vi "Text control 2 v2.3.vi"() -> ()   [LabVIEW 2016]
panel:
  out "Total lines":i32
  out "Line running":i32
  in  "byte count":u32=64
  in  "Serial Settings:Serial End Mode for Reads":u16(ring)=2 items=["None", "LastBit", "TermChar"]
  in  "Timeout (ms)":u32=10000
  in  "Enable Termination\nChar (T)":bool=TRUE
  in  "Termination char\n(0xA = '\\n' = LF)\n(0xD = '\\r' = CR)":u8=13 format="%.0x"
  in  "flow control":u16(ring) items=["None"=0, "XON/XOFF"=1, "RTS/CTS"=2, "DTR/DSR"=4]
  in  "stop bits":u16(ring)=10 items=["1.0"=10, "1.5"=15, "2.0"=20]
  in  "parity":u16(ring) items=["None", "Odd", "Even", "Mark", "Space"]
  in  "data bits":u16=8 min=5 max=8 step=1
  in  "VISA resource name":refnum<visa-resource-name>="COM6"
  in  "baud rate":u32=9600
  out "Serial output":string
  out "error out":errorcluster
  in  "Units":bool
  out "Elapsed Time":dbl caption="Elapsed Time (s)"
  out "Ion vs time":cluster{"Y data in":dbl[], "X data in":dbl[]}[](graph)
  out "Ig":dbl format="%.2e"
  out "Id":dbl format="%.2e"
  out "Is":dbl format="%.2e"
  out "I vs Vg":cluster{"Y data in":dbl[], "X data in":dbl[]}[](graph)
  in  "Panel Controls 2":T1={"Emergency Stop"=refnum, "TransGraph Max"=1e-05, "Text/Graph (text=false)"=TRUE, "TransGraph Min"=1e-11} {"TransGraph Min" format="%.2e"; "TransGraph Max" format="%.2e"}
  out "Command running:":string="#output s 0 0 0 -0.008 0.008 0.002"
  in  "Standby":T2
  in  "Full Reset":bool
  in  "SMU4":cluster{"on/off":bool, "Voltage":dbl} {"Voltage" min=-100.0 max=100.0 format="%.2f"}
  in  "Source/Drain Range":u8(slide)=6 max=11 scale=0.0..11.0
  in  "Source/Drain\nRange mode":u16(ring) items=["Auto", "Limited", "Fixed"]
  in  "Gate Range":u8(slide)=6 max=11 scale=0.0..11.0
  in  "Gate Range\nmode":u16(ring) items=["Auto", "Limited", "Fixed"]
  in  "Gate":T3={"Gate Start"=0.0, "Gate Stop"=2.0, "Gate Step (linear only)"=1.0, "Gate Compliance"=0.0001, "Gate PComp"=0.0, "Range mode"=0, "Range"=6} {"Range" max=11 scale=0.0..11.0; "Range mode" items=["Auto", "Limited", "Fixed"]; "Gate PComp" format="%^.2e"; "Gate Compliance" format="%^.2e"; "Gate Step (linear only)" format="%^.4e"; "Gate Stop" format="%^.4e"; "Gate Start" format="%^.4e"}
  in  "Drain 2":T4={"Drain Start"=0.0, "Drain Stop"=2.0, "Drain Compliance"=0.0001, "Drain Step"=1.0, "Drain PComp"=0.0, "Range mode"=0, "Range"=6} {"Range" max=11 scale=0.0..11.0; "Range mode" items=["Auto", "Limited", "Fixed"]; "Drain PComp" format="%^.2e"; "Drain Step" format="%^.4e"; "Drain Compliance" format="%^.2e"; "Drain Stop" format="%^.4e"; "Drain Start" format="%^.4e"}
  in  "Timings 2":T5={"integration time"=0, "Short/Long integration time"=0.00064, "hold time (sec)"=0.0, "delay time (sec)"=0.0, "Step Time (0 disables)"=0.0, "sweep method"=0, "Pulse period"=0.005, "Base voltage"=0.0, "Pulse width"=0.0005} {"Pulse width" min=0.0005 max=0.1 step=0.0001 format="%.4f"; "Base voltage" format="%^.4e"; "Pulse period" min=0.005 max=1.0 step=0.0001 format="%.4f"; "sweep method" items=["Continuous", "Pulsed"]; "Step Time (0 disables)" format="%.2f"; "delay time (sec)" format="%.4f"; "hold time (sec)" format="%.4f"; "Short/Long integration time" format="%^.0e"; "integration time" scale=0.0..2.0}
  in  "Panel Controls":T6={"Emergency Stop"=refnum, "TransGraph Max"=1e-05, "Text/Graph (text=false)"=TRUE} {"TransGraph Max" format="%.2e"}
  in  "Interrupt run":bool
  in  "Drain: Compliance":dbl=0.001 format="%.8f"
  in  "Gate: Compliance":dbl=0.001 format="%.8f"
  out "Path":path=path "C:/users/rlp38/09Apr2009LTtesting/test2.txt"
  in  "hold time /s":dbl format="%.2f"
  in  "delay time /s":dbl format="%.2f"
  in  "integration time":u32(slide) max=2 step=1 scale=0.0..2.0
  in  "Integration time (short)":dbl=0.0019 min=8e-05 max=0.0019 step=8e-05 format="%^.0e"
  in  "Integration time (long)":dbl=0.32 min=0.04 max=2.0 step=0.02 format="%.2f"
  in  "Step delay /s":dbl format="%.2f"
  in  "Program":string="#pulsedstressV d 0.03 20 0 0.5 0.0827 5\n#\n#itime s\n#gaterangemode l\n#drainrangemode l\n#pulsed on 0.05 0 0.02\n#transfer d 1 -1 -0.1 -1 -1 0\n#wait-min 1\n#transfer d 1 -1 -0.1 -1 -1 0\n#output d 0 -1 -0.5 0 -1 -0.1\n#transfer d -10 40 1 5 40 35\n#transfer d -10 40 1 5 40 35\n#output d 0 40 20 0 40 1\n#\n#\n#sample 1 0.008 221 6 0.003\n#samplei 400e-6 200 6 0.002 0.1\n#vsu2pulse -10 4\n#\n#stressV 0.016 0.03 2e-4 0.1e-3 11\n#stressI 220e-7 0.08 15\n#transfer s -1 1 0.5 -0.005 0.005 0.005\n#output s 0 0 0 -0.008 0.008 0.002\n"
  # "Syntax:\nitime [s|m|l]\ngaterangemode [a|l|f]\ndrainrangemode [a|l|f]\npulsed [on|off] PulsePeriod(sec) PulseBaseVoltage PulseONWidth(sec)\nstandby [on l off]\nwait NumMilliseconds\nwait-min NumMinutes\n# texthere = comment\ntransfer [s|d] VgStart VgStop VgStep VdStart VdStop VdStep\noutput [s|d] VgStart VgStop VgStep VdStart VdStop VdStep\nsample Vg Vd NumSamples Time(s) SampleInterval(s)\nsamplei Idg NumSamples Time(s) SampleInterval(s) VDGcompliance\n# if in doubt use SampleInterval(s) = 0.004\nstressV VG VD IGcompliance IDcompliance Duration(sec)\nstressI IDG VDGcompliance Duration(sec)\nvsu2pulse Bias Duration(s)\npulsedstressV [s|d] VEstop VgON VgOFF Period(s) PulseONwidth(s) Vd\nsample-fpp Vg Vd NumSamples Time\nresample-fpp Vg Vd\ntransfer-fpp [s|d] VgStart VgStop VgStep VdStart VdStop VdStep\noutput-fpp [s|d] VgStart VgStop VgStep VdStart VdStop VdStep\nserial SerialPortCommand"
  # "Time"
  # "Sec"
  # "Min"
  # "100 samples is approx 13s with medium integration"
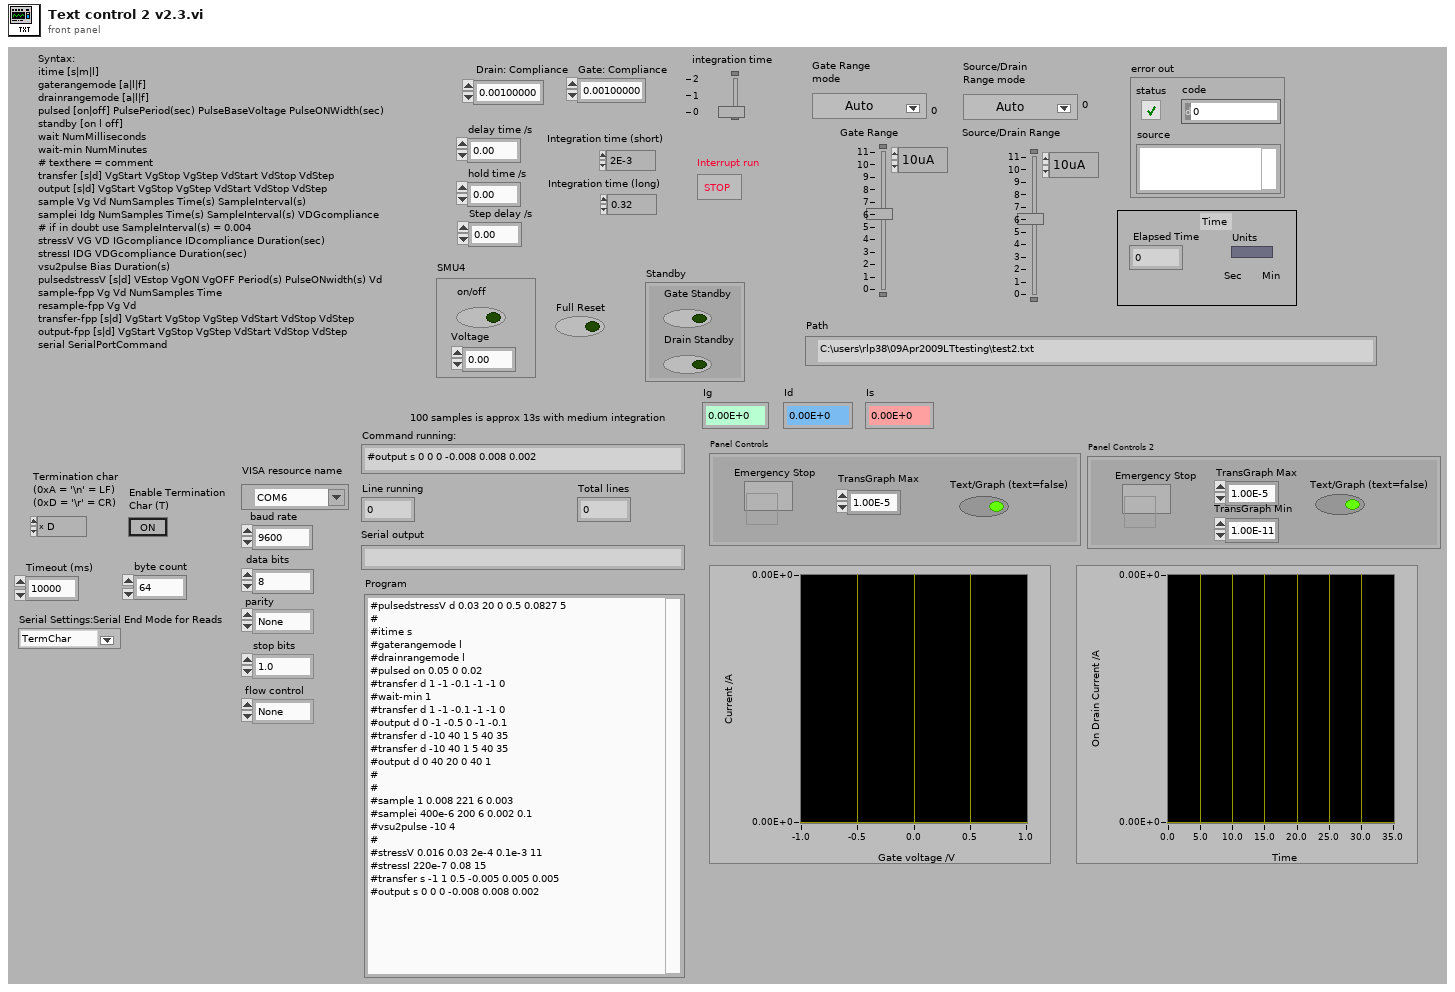
[diagram p1: front panel]
types:
  T1 = cluster{"Emergency Stop":refnum<vi>, "TransGraph Max":dbl, "Text/Graph (text=false)":bool, "TransGraph Min":dbl}
  T2 = cluster{"Gate Standby":bool, "Drain Standby":bool}
  T3 = cluster{"Gate Start":dbl, "Gate Stop":dbl, "Gate Step (linear only)":dbl, "Gate Compliance":dbl, "Gate PComp":dbl, "Range mode":u16, "Range":u8}
  T4 = cluster{"Drain Start":dbl, "Drain Stop":dbl, "Drain Compliance":dbl, "Drain Step":dbl, "Drain PComp":dbl, "Range mode":u16, "Range":u8}
  T5 = cluster{"integration time":u32, "Short/Long integration time":dbl, "hold time (sec)":dbl, "delay time (sec)":dbl, "Step Time (0 disables)":dbl, "sweep method":u16, "Pulse period":dbl, "Base voltage":dbl, "Pulse width":dbl}
  T6 = cluster{"Emergency Stop":refnum<vi>, "TransGraph Max":dbl, "Text/Graph (text=false)":bool}
  T7 = enum16{"open", "replace", "create", "open or create", "replace or create", "replace or create with confirmation"}
  T8 = cluster{"V2 Start":dbl, "V2 Step":dbl, "Number of points":i32}
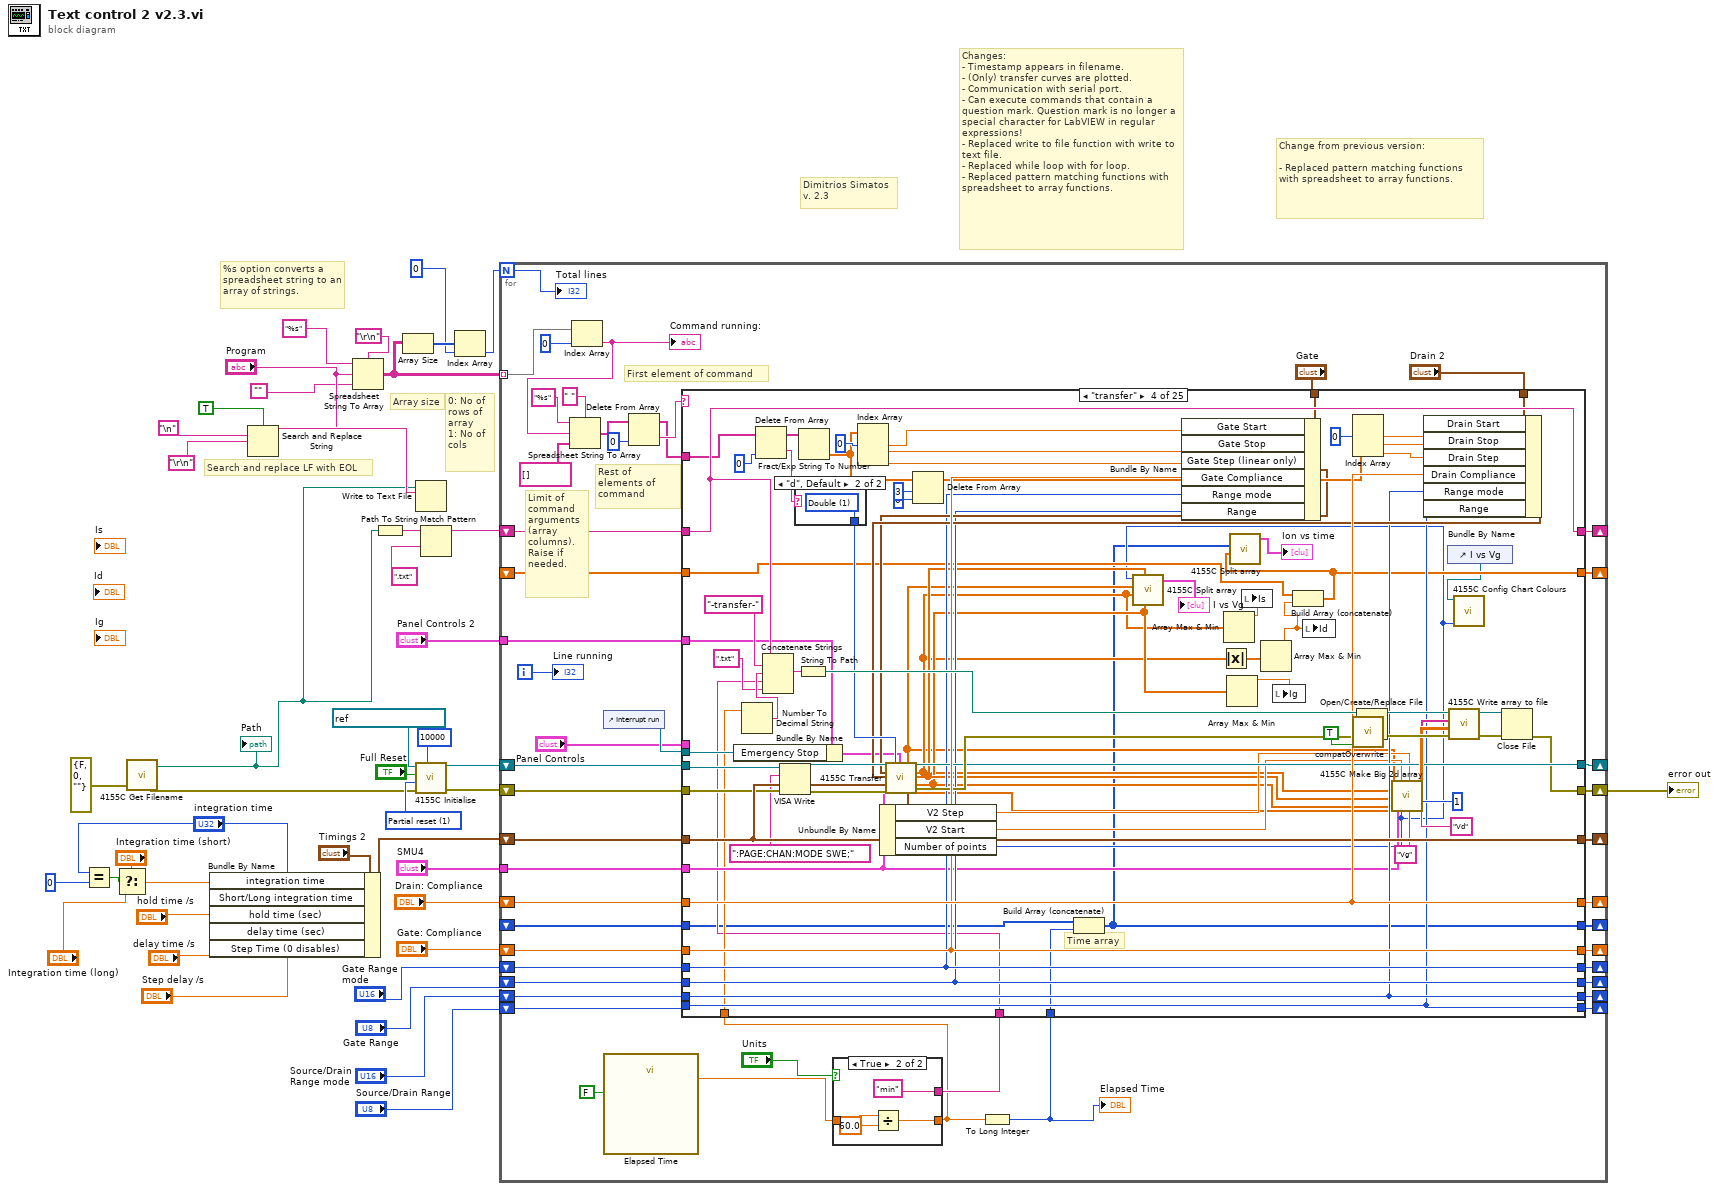
[diagram p0: block diagram]
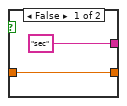
[diagram p2: hidden frame]
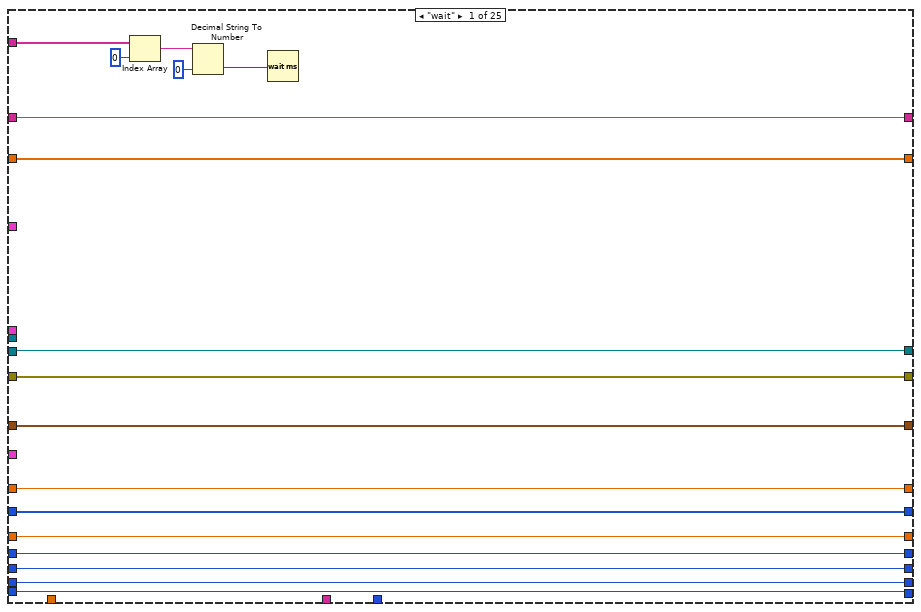
[diagram p3: hidden frame]
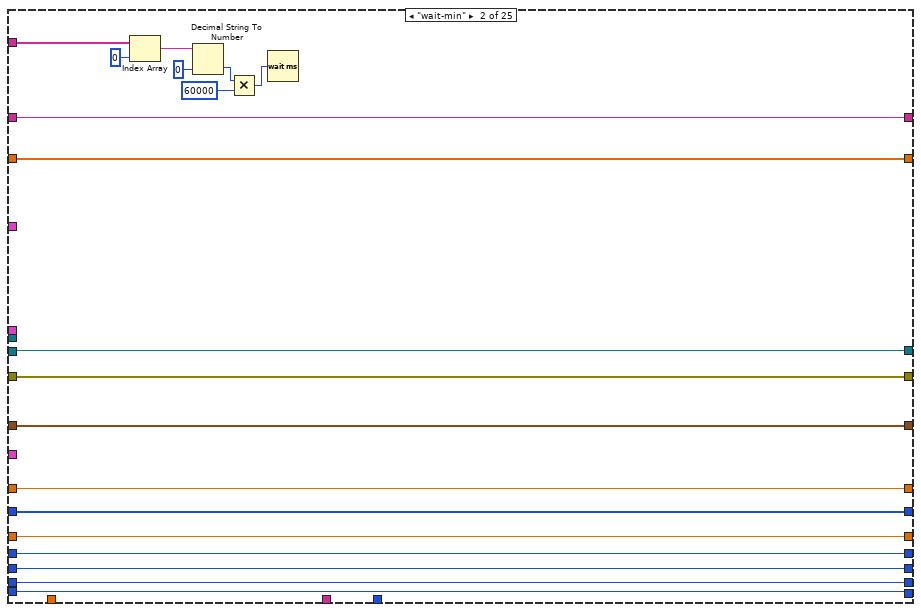
[diagram p4: hidden frame]
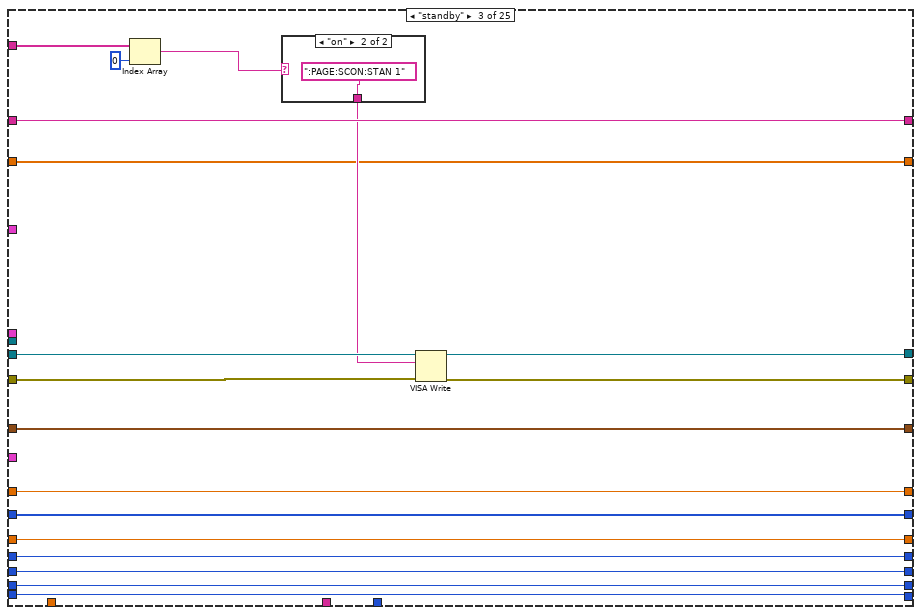
[diagram p5: hidden frame]
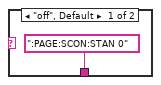
[diagram p6: hidden frame]
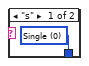
[diagram p7: hidden frame]
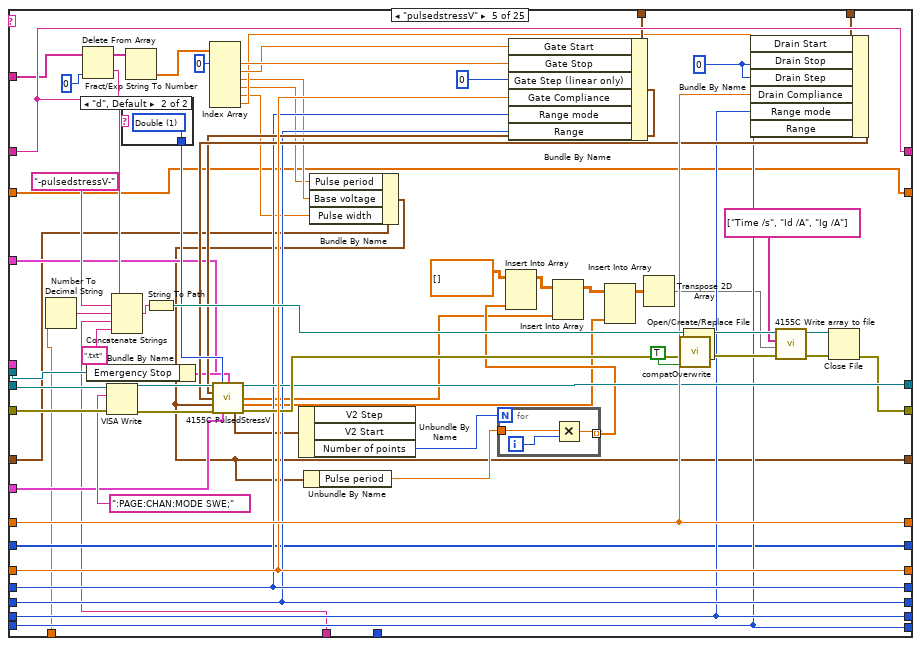
[diagram p8: hidden frame]
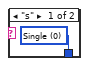
[diagram p9: hidden frame]
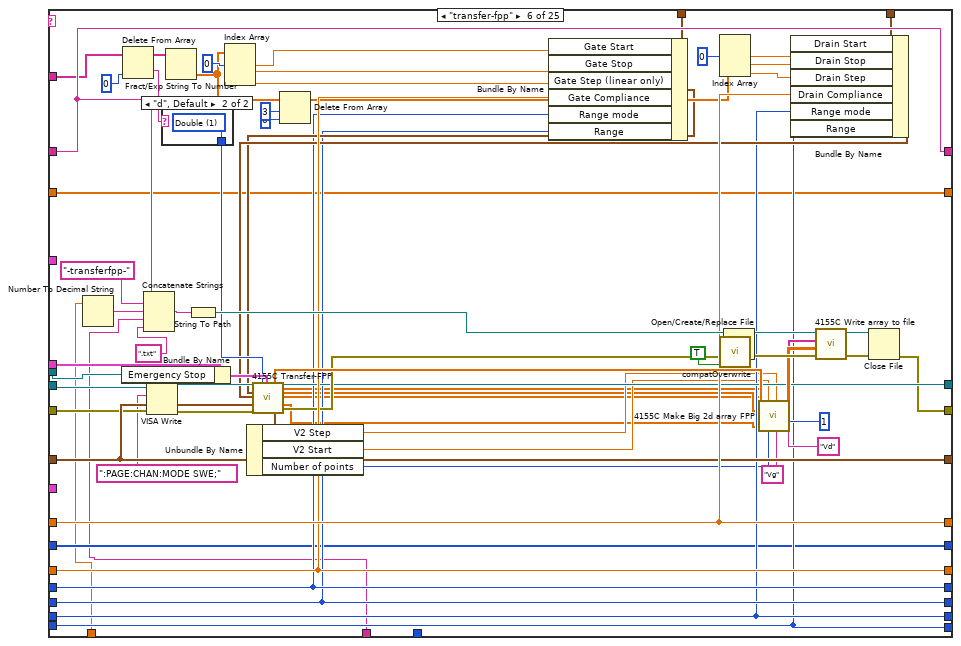
[diagram p10: hidden frame]
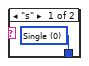
[diagram p11: hidden frame]
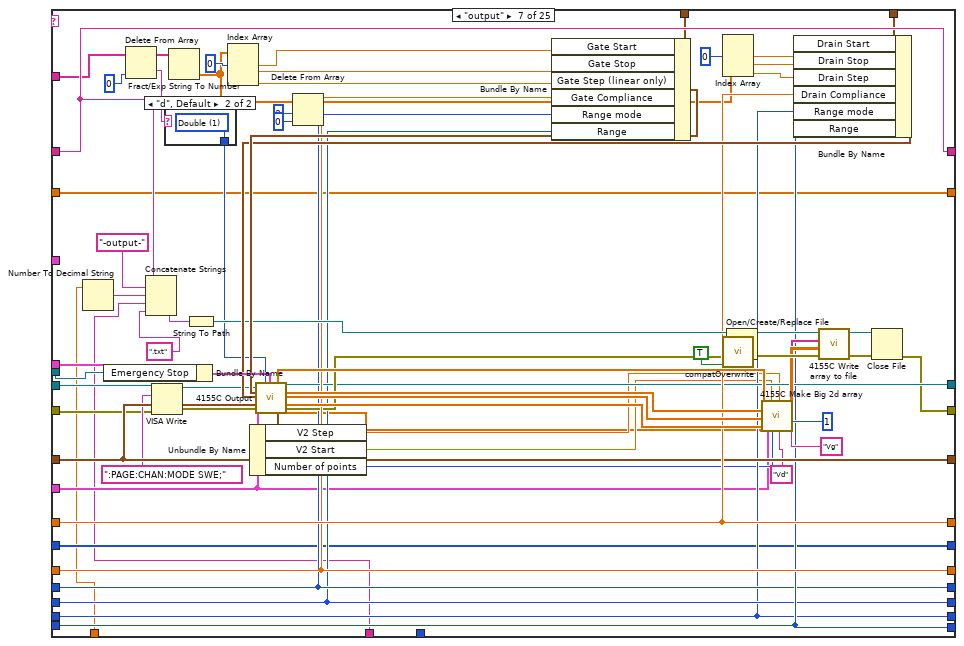
[diagram p12: hidden frame]
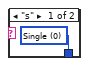
[diagram p13: hidden frame]
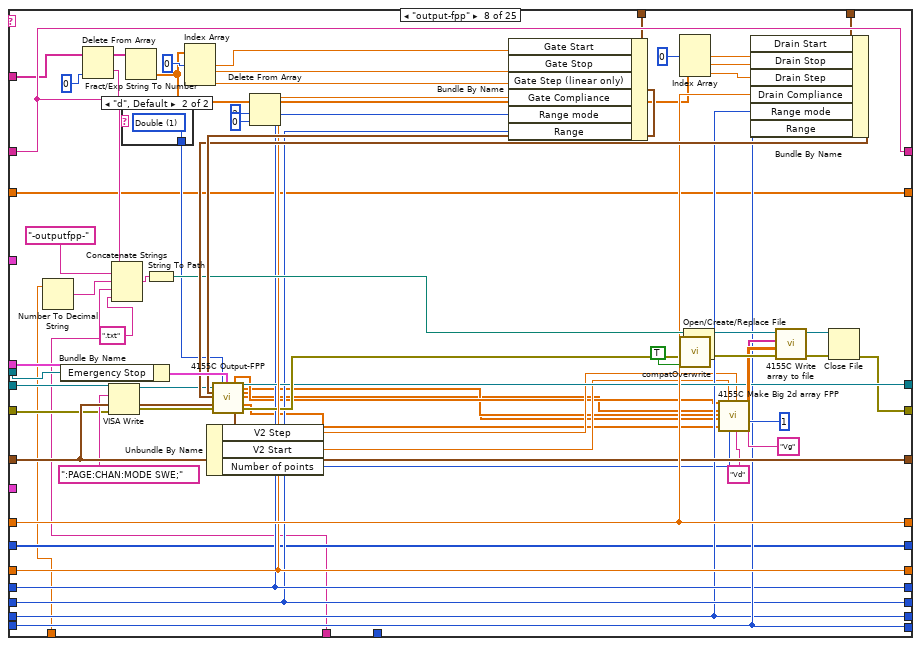
[diagram p14: hidden frame]
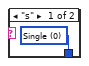
[diagram p15: hidden frame]
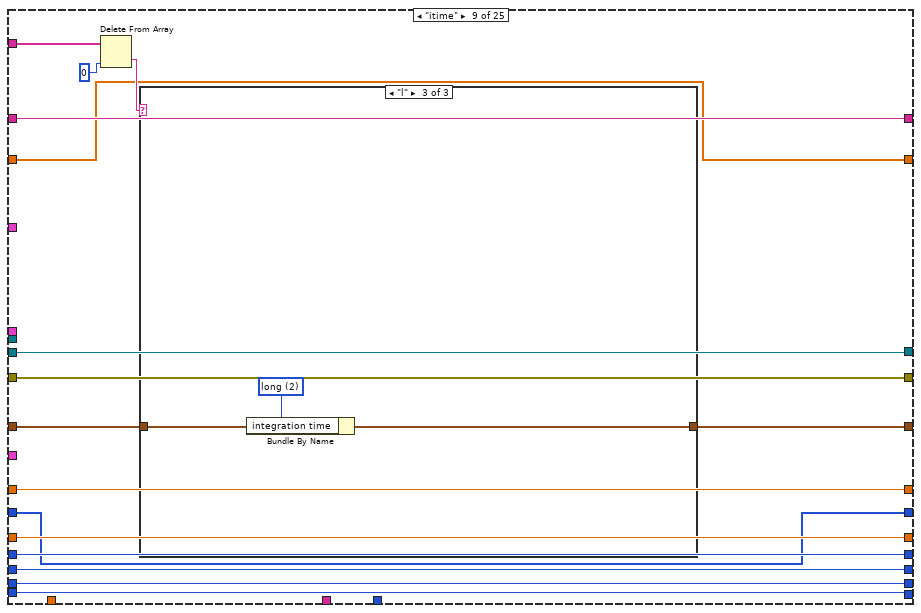
[diagram p16: hidden frame]
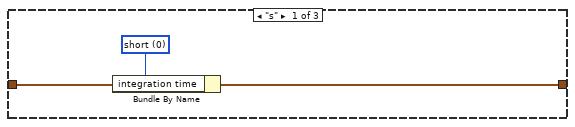
[diagram p17: hidden frame]
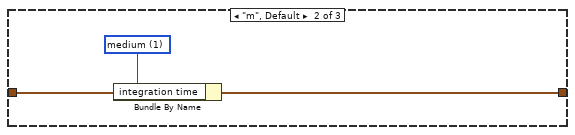
[diagram p18: hidden frame]
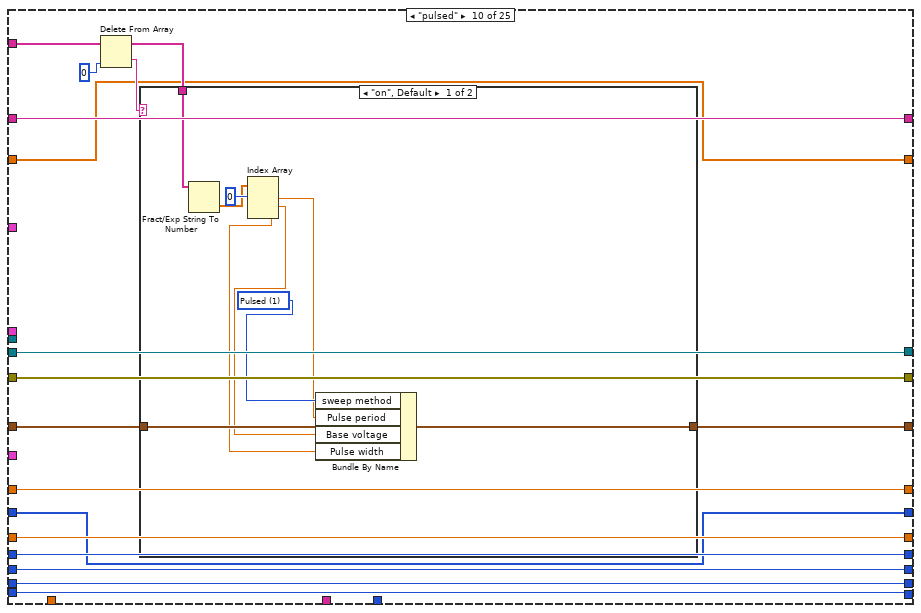
[diagram p19: hidden frame]
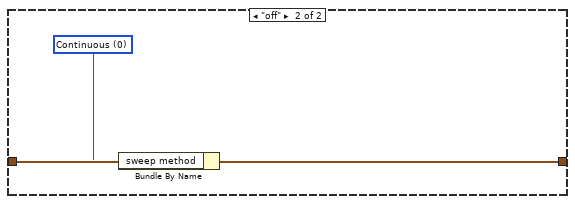
[diagram p20: hidden frame]
diagram:
  w35 = u16 1 items=["Reset All", "Partial reset"] ("Type of reset")
  # "Array size"
  # "%s option converts a spreadsheet string to an array of strings."
  # "0: No of rows of array\n1: No of cols"
  # "Change from previous version:\n\n- Replaced pattern matching functions with spreadsheet to array functions."
  # "Dimitrios Simatos\nv. 2.3"
  # "Changes:\n- Timestamp appears in filename.\n- (Only) transfer curves are plotted.\n- Communication with serial port.\n- Can execute commands that contain a question mark. Question mark is no longer a special character for LabVIEW in regular expressions!\n- Replaced write to file function with write to text file.\n- Replaced while loop with for loop.\n- Replaced pattern matching functions with spreadsheet to array functions."
  # "Search and replace LF with EOL"
  n1 = Equal?(x="integration time", y=u32 0) -> (x = y?=w39:bool)
  n2 = Select(t="Integration time (short)", s=w39, f="Integration time (long)") -> (s? t:f=w43:dbl)
  n3 = call "4155C Get Filename.vi"("error in (no error)"=errorcluster {"status"=FALSE, "code"=0, "source"=""}) -> ("error out"=w30:errorcluster, "path"=w1:path)  [unwired: 2 in, 1 out]
  "Path" <- w1
  n4 = Bundle By Name(cluster="Timings 2", "integration time"="integration time", "Short/Long integration time"=w43, "hold time (sec)"="hold time /s", "delay time (sec)"="delay time /s", "Step Time (0 disables)"="Step delay /s") -> (w27:T5)
  n5 = Search and Replace String(replace all?=TRUE ("replace all? (F)"), input string="Program", search string="\n", replace string="\r\n") -> (result string=w17:string)  [unwired: 4 in, 3 out]
  n6 = Spreadsheet String To Array(delimiter (Tab)="\r\n", format string="%s", spreadsheet string="Program", array type (2D Dbl)="") -> (array=w7:string[][])
  n7 = Path To String(path=w1) -> (string=w4:string)
  n8 = Array Size(array=w7) -> (size(s)=w11:i32[])
  n9 = Write to Text File(file (use dialog)=w1, text=w17) -> ()  [unwired: 2 in, 3 out]
  n10 = call "4155C Initialise.vi"("VISA resource name in"=refnum<visa-resource-name> "GPIB0::14::INSTR", "Reset"="Full Reset", "Type of reset"=w35, "error in (no error)"=w30, "VISA Timeout Value"=u32 10000) -> ("VISA Resource Name out"=w29:refnum<visa-resource-name>, "error out"=w28:errorcluster)
  n11 = Match Pattern(string=w4, regular expression=".txt") -> (before substring=w2:string)  [unwired: 1 in, 3 out]
  n12 = Index Array(array=w11, index=0) -> (element=w9:i32)
  n13 = for {
    N: w9 -> [w53]
    tunnel: "SMU4" -> [w68]
    shift-left: "Source/Drain Range" -> [w73]
    shift-right: [w69] -> _
    shift-left: "Source/Drain\nRange mode" -> [w74]
    shift-right: [w70] -> _
    shift-left: "Gate Range" -> [w75]
    shift-right: [w71] -> _
    shift-left: "Gate Range\nmode" -> [w76]
    shift-right: [w72] -> _
    shift-left: "Gate: Compliance" -> [w87]
    shift-right: [w82] -> _
    shift-left: "Drain: Compliance" -> [w88]
    shift-right: [w83] -> _
    shift-left: w27 -> [w89]
    shift-right: [w84] -> _
    shift-left: w28 -> [w90]
    shift-right: [w85] -> w13
    shift-left: w29 -> [w91]
    shift-right: [w86] -> _
    shift-left: w2 -> [w92]
    shift-right: [w81] -> _
    tunnel: "Panel Controls 2" -> [w67]
    shift-right: [w66] -> _
    shift-left: _ -> [w65]
    shift-right: [w60] -> _
    shift-left: _ -> [w59]
    tunnel: w7 -> [w56] mode=indexing
    i -> [w54]
    # "Limit of command arguments (array columns). Raise if needed."
    # "Rest of elements of command"
    # "First element of command"
    n14 = Index Array(array=w56, index=0 ("line index")) -> (element=w49:string)
    "Command running:" <- w49
    n15 = Spreadsheet String To Array(delimiter (Tab)=" ", format string="%s", spreadsheet string=w49, array type (2D Dbl)=string[] []) -> (array=w46:string[])
    n16 = control-ref of="Interrupt run"() -> (w80:refnum<vi>)
    n17 = call "Elapsed Time"("Auto Reset"=FALSE) -> ("Elapsed Time (s)"=w61:dbl)  [unwired: 11 in, 7 out]
    n18 = Delete From Array(array=w46, index=0) -> (deleted portion=w47:string, array with subset deleted=w45:string[])  [unwired: 1 in]
    n19 = case shown="True" "Units" {
      tunnel: ["sec" "min"] -> w62
      tunnel: [w93 w97] -> w58
      tunnel: w61 -> [w93 w96]
      frame False {
      }
      frame True {
        n20 = Divide(x=w96, y=60.0) -> (x/y=w97:dbl)
      }
    }
    n21 = To Long Integer(number=w58) -> (32bit integer=w57:i32)
    "Elapsed Time" <- w57
    n22 = case shown="\"transfer\"" w47 {
      tunnel: w45 -> [w115 w134 w152 w216 w287 w356 w423 w498 w536 w562 w589 w614 w635 w649 _ _ w753 w814 _ w879 w923 w965 w1035 w1097 w1104]
      tunnel: w92 -> [w110 w130 w150 w224 w294 w364 w431 w506 w525 w551 w581 w607 w629 w642 w661 w703 w731 w796 w827 w866 w910 w953 w1029 w1093 w1106]
      tunnel: w91 -> [w109 w129 w141 w194 w278 w333 w399 w474 w526 w552 w582 w608 w630 w643 w666 w705 w759 w820 w831 w885 w929 w971 w1041 w1051 w1110]
      tunnel: w90 -> [w108 w128 w140 w193 w277 w332 w396 w471 w527 w553 w583 w609 w631 w644 w665 w676 w758 w819 w830 w884 w928 w970 w1040 w1050 w1109]
      tunnel: w89 -> [w107 w127 w149 w220 w253 w360 w427 w502 w535 w561 w580 w606 w628 w641 w664 w700 w722 w788 w836 w859 w903 w946 w1028 w1092 w1111]
      tunnel: w88 -> [w106 w126 w148 w222 w292 w362 w429 w504 w534 w560 w588 w613 w634 w648 w663 w685 w757 w818 w839 w883 w927 w969 w1039 w1101 w1112]
      tunnel: w87 -> [w105 w125 w147 w221 w291 w361 w428 w503 w533 w559 w587 w612 w633 w647 w662 w686 w732 w797 w838 w867 w911 w954 w1030 w1094 w1114]
      tunnel: [w109 w129 w139 w218 w289 w358 w425 w500 w526 w552 w582 w608 w630 w643 w666 w705 w723 w770 w829 w860 w904 w947 w981 w1053 w1110] -> w86
      tunnel: [w108 w128 w138 w217 w288 w357 w424 w499 w527 w553 w583 w609 w631 w644 w665 w675 w733 w771 w828 w868 w912 w955 w980 w1052 w1108] -> w85
      tunnel: [w107 w127 w149 w220 w249 w360 w427 w502 w528 w554 w580 w606 w628 w641 w664 w700 w722 w788 w836 w859 w903 w946 w1028 w1092 w1111] -> w84
      tunnel: [w106 w126 w148 w222 w292 w362 w429 w504 w534 w560 w588 w613 w634 w648 w663 w685 w757 w818 w839 w883 w927 w969 w1039 w1101 w1112] -> w83
      tunnel: [w105 w125 w147 w221 w291 w361 w428 w503 w533 w559 w587 w612 w633 w647 w662 w686 w732 w797 w838 w867 w911 w954 w1030 w1094 w1114] -> w82
      tunnel: [w110 w130 w150 w224 w294 w364 w431 w506 w525 w551 w581 w607 w629 w642 w661 w703 w731 w796 w827 w866 w910 w953 w1029 w1093 w1106] -> w81
      tunnel: w80 -> [_ _ _ w227 w298 w369 w439 w510 _ _ _ _ _ _ _ _ w728 w793 _ w865 w909 w952 w1001 w1069 _]
      tunnel: "Gate" -> [_ _ _ w203 w281 w343 w410 w485 _ _ _ _ _ _ _ _ _ _ _ _ _ _ _ _ _]
      tunnel: "Drain 2" -> [_ _ _ w202 w280 w342 w409 w484 _ _ _ _ _ _ _ _ _ _ _ _ _ _ _ _ _]
      tunnel: "Panel Controls" -> [_ _ _ _ _ w341 w408 w483 _ _ _ _ _ _ _ _ _ _ _ _ _ _ _ _ _]
      tunnel: w76 -> [w104 w124 w146 w187 w271 w326 w394 w469 w532 w558 _ w605 w627 w640 w660 w687 w718 w784 w832 w855 w899 w942 w1024 w1088 w1115]
      tunnel: w75 -> [w103 w123 w145 w186 w270 w325 w393 w468 w531 w557 w586 _ w618 w646 w659 w688 w719 w785 w833 w856 w900 w943 w1025 w1089 w1116]
      tunnel: w74 -> [w102 w122 w144 w185 w269 w324 w392 w467 w530 w556 w585 w611 w632 _ w658 w689 w720 w786 w834 w857 w901 w944 w1026 w1090 w1117]
      tunnel: w73 -> [w101 w121 w143 w184 w268 w323 w395 w470 w529 w555 w584 w610 _ w645 w657 w690 w721 w787 w835 w858 w902 w945 w1027 w1091 w1118]
      tunnel: [w104 w124 w146 w187 w271 w326 w394 w469 w532 w558 w579 w605 w627 w640 w660 w687 w718 w784 w832 w855 w899 w942 w1024 w1088 w1115] -> w72
      tunnel: [w103 w123 w145 w186 w270 w325 w393 w468 w531 w557 w586 w597 w618 w646 w659 w688 w719 w785 w833 w856 w900 w943 w1025 w1089 w1116] -> w71
      tunnel: [w102 w122 w144 w185 w269 w324 w392 w467 w530 w556 w585 w611 w632 w639 w658 w689 w720 w786 w834 w857 w901 w944 w1026 w1090 w1117] -> w70
      tunnel: [w101 w121 w143 w184 w268 w323 w395 w470 w529 w555 w584 w610 w619 w645 w657 w690 w721 w787 w835 w858 w902 w945 w1027 w1091 w1118] -> w69
      tunnel: w68 -> [_ _ _ w179 w265 _ w387 _ _ _ _ _ _ _ _ _ _ _ _ _ _ _ _ _ _]
      tunnel: w67 -> [_ _ _ w177 w264 _ _ _ _ _ _ _ _ _ _ _ _ _ _ _ _ _ _ _ _]
      tunnel: [w100 w117 w136 w166 w241 w313 w384 w456 w524 w549 w578 w596 w617 w638 w656 w671 w710 w768 w826 w844 w892 w936 w978 w1046 w1107] -> w66
      tunnel: w65 -> [w100 w117 w136 w165 w241 w313 w384 w456 w524 w549 w578 w596 w617 w638 w656 w671 w710 w768 w826 w844 w892 w936 w978 w1046 w1107]
      tunnel: w58 -> [_ _ _ w161 w238 w311 w381 w453 _ _ _ _ _ _ _ w669 w708 w765 _ w841 w889 w933 w975 w1042 _]
      tunnel: w62 -> [_ _ _ w158 w237 w309 w380 w452 _ _ _ _ _ _ _ w667 w706 w764 _ w840 w888 w932 w974 w1043 _]
      tunnel: w57 -> [_ _ _ w155 _ _ _ _ _ _ _ _ _ _ _ _ _ _ _ _ _ _ _ _ _]
      tunnel: [w99 w116 w135 w157 w240 w312 w383 w455 w523 w548 w577 w595 w616 w637 w655 w670 w709 w767 w825 w843 w891 w935 w977 w1045 w1113] -> w60
      tunnel: w59 -> [w99 w116 w135 w156 w240 w312 w383 w455 w523 w548 w577 w595 w616 w637 w655 w670 w709 w767 w825 w843 w891 w935 w977 w1045 w1113]
      frame "wait" {
        n23 = Index Array(array=w115, index=0 ("Index")) -> (element=w113:string)
        n24 = Decimal String To Number(string=w113, default (0L)=u32 0) -> (number=w112:u32)  [unwired: 1 in, 1 out]
        n25 = Wait (ms)(milliseconds to wait=w112) -> ()  [unwired: 1 out]
      }
      frame "wait-min" {
        n26 = Index Array(array=w134, index=0 ("Index")) -> (element=w132:string)
        n27 = Decimal String To Number(string=w132, default (0L)=u32 0) -> (number=w120:u32)  [unwired: 1 in, 1 out]
        n28 = Multiply(x=w120, y=u32 60000) -> (x*y=w119:u32)
        n29 = Wait (ms)(milliseconds to wait=w119) -> ()  [unwired: 1 out]
      }
      frame "standby" {
        n30 = Index Array(array=w152, index=0 ("Index")) -> (element=w142:string)
        n31 = case shown="\"on\"" w142 {
          tunnel: [":PAGE:SCON:STAN 0" ":PAGE:SCON:STAN 1"] -> w137
          frame "off", Default {
          }
          frame "on" {
          }
        }
        n32 = VISA Write(VISA resource name=w141, write buffer=w137, error in (no error)=w140) -> (VISA resource name out=w139:refnum<visa-resource-name>, error out=w138:errorcluster)  [unwired: 1 out]
      }
      frame "transfer" {
        # "Time array"
        n33 = Bundle By Name(cluster=w177, "Emergency Stop"=w227) -> (w178:T1)
        n34 = Number To Decimal String(number=w161) -> (decimal integer string=w160:string)  [unwired: 1 in]
        n35 = Delete From Array(array=w216, index=0 ("Index")) -> (deleted portion=w214:string, array with subset deleted=w213:string[])  [unwired: 1 in]
        n36 = Concatenate Strings(w224, "-transfer-" ("Prefix"), w160, w158, ".txt" ("Suffix")) -> (w226:string)
        n37 = VISA Write(VISA resource name=w194, write buffer=":PAGE:CHAN:MODE SWE;" ("write buffer (\"\")"), error in (no error)=w193) -> (VISA resource name out=w191:refnum<visa-resource-name>, error out=w192:errorcluster)  [unwired: 1 out]
        n38 = case shown="\"d\", Default" w214 {
          tunnel: [w235 w236] -> w212
          frame "s" {
            w235 = u16 0 items=["Single", "Double"] ("sweep mode")
          }
          frame "d", Default {
            w236 = u16 1 items=["Single", "Double"] ("sweep mode")
          }
        }
        n39 = String To Path(string=w226) -> (path=w223:path)
        n40 = Fract/Exp String To Number(string=w213) -> (number=w198:dbl[])  [unwired: 3 in, 1 out]
        n41 = Index Array(array=w198, index #1=0 ("Index")) -> (element #1=w211:dbl, element #2=w210:dbl, element #3=w209:dbl)  [unwired: 2 in]
        n42 = Delete From Array(array=w198, length=3 ("Length"), index=0 ("Index")) -> (array with subset deleted=w196:dbl[])  [unwired: 1 out]
        n43 = Build Array (concatenate)(w156, w155) -> (w157:i32[])
        n44 = Bundle By Name(cluster=w203, "Gate Start"=w211, "Gate Stop"=w210, "Gate Step (linear only)"=w209, "Gate Compliance"=w221, "Range mode"=w187, "Range"=w186) -> (w188:T3)
        n45 = Index Array(array=w196, index #1=0 ("Index")) -> (element #1=w206:dbl, element #2=w205:dbl, element #3=w204:dbl)  [unwired: 2 in]
        n46 = call <vilib>:"compatOverwrite.vi"("overwrite (F)"=TRUE) -> ("overwrite?"=w176:T7)
        n47 = Bundle By Name(cluster=w202, "Drain Start"=w206, "Drain Stop"=w205, "Drain Step"=w204, "Drain Compliance"=w222, "Range mode"=w185, "Range"=w184) -> (w189:T4)
        n48 = call "4155C Transfer.vi"("VISA resource name in"=w191, "Gate"=w188, "Drain"=w189, "Timings"=w220, "error in (no error)"=w192, "SMU4"=w179, "sweep mode"=w212, "Panel Controls"=w178) -> ("VG"=w167:dbl[], "Outparams"=w183:T8, "VISA Resource Name out"=w218:refnum<visa-resource-name>, "IS"=w169:dbl[], "ID"=w174:dbl[], "IG"=w170:dbl[], "error out"=w219:errorcluster, "SMU4"=w180:dbl[])  [unwired: 12 in]
        n49 = Unbundle By Name(w183) -> ("V2 Step"=w182:dbl, "V2 Start"=w181:dbl, "Number of points"=w163:i32)
        n50 = call "4155C Split array.vi"("Number of VAR2 steps"=w163, "Y2 data in"=w174, "X data in"=w167, "Y1 data in"=w169, "Y3 data in"=w170) -> ("Array of clusters"=→"I vs Vg":cluster{"Y data in":dbl[], "X data in":dbl[]}[])  [unwired: 2 in, 1 out]
        n51 = Absolute Value(x=w169) -> (abs(x)=w173:dbl[])
        n52 = Array Max & Min(array=w169) -> (max value=w171:dbl)  [unwired: 3 out]
        n53 = Array Max & Min(array=w170) -> (max value=w172:dbl)  [unwired: 3 out]
        n54 = local write "Is"(w171) -> ()
        n55 = Array Max & Min(array=w173) -> (max value=w164:dbl)  [unwired: 3 out]
        n56 = local write "Ig"(w172) -> ()
        n57 = Build Array (concatenate)(w165, w164) -> (w166:dbl[])
        n58 = call "4155C Split array.vi"("X data in"=w157, "Y1 data in"=w166) -> ("Array of clusters"=→"Ion vs time":cluster{"Y data in":dbl[], "X data in":dbl[]}[])  [unwired: 5 in, 1 out]
        n59 = local write "Id"(w164) -> ()
        n60 = Open/Create/Replace File(file path (use dialog)=w223, error in=w219, operation (0:open)=w176) -> (refnum out=w232:refnum<file>, error out=w233:errorcluster)  [unwired: 3 in, 1 out]
        n61 = call "4155C Make Big 2d array.vi"("1D Var1"=w167, "1d IS"=w169, "1d ID"=w174, "1d IG"=w170, "1d SMU4"=w180, "SMU4"=w179, "VAR2 START"=w181, "Number of VAR2 steps"=w163, "VAR2 STEP"=w182, "VAR1 Name"="Vg", "Decimal places in header"=i8 1, "VAR2 Name"="Vd") -> ("Header array"=w228:string[], "Data array"=w229:dbl[][])  [unwired: 14 in]
        n62 = control-ref of="I vs Vg"() -> (w162:refnum<vi>)
        n63 = call "4155C Write array to file.vi"("Byte Stream File Refnum"=w232, "Header"=w228, "Data Array"=w229, "error in (no error)"=w233) -> ("dup refnum"=w230:refnum<file>, "error out"=w231:errorcluster)  [unwired: 1 in]
        n64 = call "4155C Config Chart Colours.vi"("Numeric"=w163, "XY Graph 2"=w162) -> ()  [unwired: 6 in]
        n65 = Close File(refnum=w230, error in=w231) -> (error out=w217:errorcluster)  [unwired: 1 out]
      }
      frame "pulsedstressV" {
        w247 = 0
        n66 = Number To Decimal String(number=w238) -> (decimal integer string=w295:string)  [unwired: 1 in]
        n67 = Delete From Array(array=w287, index=0 ("Index")) -> (deleted portion=w285:string, array with subset deleted=w284:string[])  [unwired: 1 in]
        n68 = Bundle By Name(cluster=w264, "Emergency Stop"=w298) -> (w266:T1)
        n69 = VISA Write(VISA resource name=w278, write buffer=":PAGE:CHAN:MODE SWE;" ("write buffer (\"\")"), error in (no error)=w277) -> (VISA resource name out=w275:refnum<visa-resource-name>, error out=w276:errorcluster)  [unwired: 1 out]
        n70 = Concatenate Strings(w294, "-pulsedstressV-" ("Substring"), w295, w237, ".txt" ("Substring")) -> (w297:string)
        n71 = case shown="\"d\", Default" w285 {
          tunnel: [w307 w308] -> w283
          frame "s" {
            w307 = u16 0 items=["Single", "Double"] ("sweep mode")
          }
          frame "d", Default {
            w308 = u16 1 items=["Single", "Double"] ("sweep mode")
          }
        }
        n72 = Fract/Exp String To Number(string=w284) -> (number=w279:dbl[])  [unwired: 3 in, 1 out]
        n73 = String To Path(string=w297) -> (path=w293:path)
        n74 = Index Array(array=w279, index #1=0 ("Index")) -> (element #1=w256:dbl, element #2=w255:dbl, element #3=w252:dbl, element #4=w251:dbl, element #5=w250:dbl, element #6=w254:dbl)  [unwired: 5 in]
        n75 = Bundle By Name(cluster=w253, "Pulse period"=w251, "Base voltage"=w252, "Pulse width"=w250) -> (w249:T5)
        n76 = Unbundle By Name(w249) -> ("Pulse period"=w257:dbl)
        n77 = Bundle By Name(cluster=w281, "Gate Start"=w255, "Gate Stop"=w256, "Gate Step (linear only)"=0, "Gate Compliance"=w291, "Range mode"=w271, "Range"=w270) -> (w272:T3)
        n78 = call <vilib>:"compatOverwrite.vi"("overwrite (F)"=TRUE) -> ("overwrite?"=w242:T7)
        n79 = Bundle By Name(cluster=w280, "Drain Start"=w254, "Drain Stop"=w247, "Drain Step"=w247, "Drain Compliance"=w292, "Range mode"=w269, "Range"=w268) -> (w273:T4)
        n80 = call "4155C PulsedStressV.vi"("VISA resource name in"=w275, "sweep mode"=w283, "Panel Controls"=w266, "Gate"=w272, "Drain"=w273, "Timings"=w249, "error in (no error)"=w276, "SMU4"=w265) -> ("VISA Resource Name out"=w289:refnum<visa-resource-name>, "ID"=w245:dbl[], "IG"=w243:dbl[], "Outparams"=w267:T8, "error out"=w290:errorcluster)  [unwired: 3 in]
        n81 = Unbundle By Name(w267) -> ("Number of points"=w244:i32)  [unwired: 2 out]
        n82 = for {
          N: w244 -> [_]
          tunnel: [w304] -> w246 mode=indexing
          tunnel: w257 -> [w306]
          i -> [w305]
          n83 = Multiply(x=w306, y=w305) -> (x*y=w304:dbl)
        }
        n84 = Insert Into Array(array=dbl[][] [] ("Input Array"), new element=w246) -> (w258:dbl[][])  [unwired: 2 in]
        n85 = Insert Into Array(array=w258, new element=w245) -> (w263:dbl[][])  [unwired: 2 in]
        n86 = Insert Into Array(array=w263, new element=w243) -> (w262:dbl[][])  [unwired: 2 in]
        n87 = Transpose 2D Array(2D array=w262) -> (transposed array=w261:dbl[][])
        n88 = Open/Create/Replace File(file path (use dialog)=w293, error in=w290, operation (0:open)=w242) -> (refnum out=w301:refnum<file>, error out=w302:errorcluster)  [unwired: 3 in, 1 out]
        n89 = call "4155C Write array to file.vi"("Byte Stream File Refnum"=w301, "Header"=string[] ["Time /s", "Id /A", "Ig /A"], "Data Array"=w261, "error in (no error)"=w302) -> ("dup refnum"=w299:refnum<file>, "error out"=w300:errorcluster)  [unwired: 1 in]
        n90 = Close File(refnum=w299, error in=w300) -> (error out=w288:errorcluster)  [unwired: 1 out]
      }
      frame "transfer-fpp" {
        n91 = Number To Decimal String(number=w311) -> (decimal integer string=w365:string)  [unwired: 1 in]
        n92 = Bundle By Name(cluster=w341, "Emergency Stop"=w369) -> (w377:T6)
        n93 = Delete From Array(array=w356, index=0 ("Index")) -> (deleted portion=w354:string, array with subset deleted=w353:string[])  [unwired: 1 in]
        n94 = Concatenate Strings(w364, "-transferfpp-" ("Substring"), w365, w309, ".txt" ("Substring")) -> (w367:string)
        n95 = VISA Write(VISA resource name=w333, write buffer=":PAGE:CHAN:MODE SWE;" ("write buffer (\"\")"), error in (no error)=w332) -> (VISA resource name out=w330:refnum<visa-resource-name>, error out=w331:errorcluster)  [unwired: 1 out]
        n96 = case shown="\"d\", Default" w354 {
          tunnel: [w378 w379] -> w352
          frame "s" {
            w378 = u16 0 items=["Single", "Double"] ("sweep mode")
          }
          frame "d", Default {
            w379 = u16 1 items=["Single", "Double"] ("sweep mode")
          }
        }
        n97 = Fract/Exp String To Number(string=w353) -> (number=w337:dbl[])  [unwired: 3 in, 1 out]
        n98 = String To Path(string=w367) -> (path=w363:path)
        n99 = Index Array(array=w337, index #1=0 ("Index")) -> (element #1=w351:dbl, element #2=w350:dbl, element #3=w349:dbl)  [unwired: 2 in]
        n100 = Delete From Array(array=w337, length=3 ("Length"), index=0 ("Index")) -> (array with subset deleted=w335:dbl[])  [unwired: 1 out]
        n101 = Bundle By Name(cluster=w343, "Gate Start"=w351, "Gate Stop"=w350, "Gate Step (linear only)"=w349, "Gate Compliance"=w361, "Range mode"=w326, "Range"=w325) -> (w327:T3)
        n102 = Index Array(array=w335, index #1=0 ("Index")) -> (element #1=w346:dbl, element #2=w345:dbl, element #3=w344:dbl)  [unwired: 2 in]
        n103 = call <vilib>:"compatOverwrite.vi"("overwrite (F)"=TRUE) -> ("overwrite?"=w314:T7)
        n104 = Bundle By Name(cluster=w342, "Drain Start"=w346, "Drain Stop"=w345, "Drain Step"=w344, "Drain Compliance"=w362, "Range mode"=w324, "Range"=w323) -> (w328:T4)
        n105 = call "4155C Transfer-FPP.vi"("VISA resource name in"=w330, "Gate"=w327, "Drain"=w328, "Timings"=w360, "error in (no error)"=w331, "sweep mode"=w352, "Panel Controls"=w377) -> ("VG"=w368:dbl[], "Outparams"=w322:T8, "VISA Resource Name out"=w358:refnum<visa-resource-name>, "Vprobe2"=w318:dbl[], "ID"=w317:dbl[], "IG"=w316:dbl[], "Vprobe1"=w315:dbl[], "error out"=w359:errorcluster)  [unwired: 13 in]
        n106 = Unbundle By Name(w322) -> ("V2 Step"=w321:dbl, "V2 Start"=w320:dbl, "Number of points"=w319:i32)
        n107 = Open/Create/Replace File(file path (use dialog)=w363, error in=w359, operation (0:open)=w314) -> (refnum out=w374:refnum<file>, error out=w375:errorcluster)  [unwired: 3 in, 1 out]
        n108 = call "4155C Make Big 2d array FPP.vi"("1D Var1"=w368, "1d ID"=w317, "1d Vp2"=w318, "1d IG"=w316, "1d Vp1"=w315, "VAR2 START"=w320, "Number of VAR2 steps"=w319, "VAR2 STEP"=w321, "VAR1 Name"="Vg", "Decimal places in header"=i8 1, "VAR2 Name"="Vd") -> ("Header array"=w370:string[], "Data array"=w371:dbl[][])  [unwired: 15 in]
        n109 = call "4155C Write array to file.vi"("Byte Stream File Refnum"=w374, "Header"=w370, "Data Array"=w371, "error in (no error)"=w375) -> ("dup refnum"=w372:refnum<file>, "error out"=w373:errorcluster)  [unwired: 1 in]
        n110 = Close File(refnum=w372, error in=w373) -> (error out=w357:errorcluster)  [unwired: 1 out]
      }
      frame "output" {
        n111 = Number To Decimal String(number=w381) -> (decimal integer string=w432:string)  [unwired: 1 in]
        n112 = Bundle By Name(cluster=w408, "Emergency Stop"=w439) -> (w449:T6)
        n113 = Delete From Array(array=w423, index=0 ("Index")) -> (deleted portion=w421:string, array with subset deleted=w420:string[])  [unwired: 1 in]
        n114 = Concatenate Strings(w431, "-output-" ("Substring"), w432, w380, ".txt" ("Substring")) -> (w434:string)
        n115 = VISA Write(VISA resource name=w399, write buffer=":PAGE:CHAN:MODE SWE;" ("write buffer (\"\")"), error in (no error)=w396) -> (VISA resource name out=w398:refnum<visa-resource-name>, error out=w397:errorcluster)  [unwired: 1 out]
        n116 = case shown="\"d\", Default" w421 {
          tunnel: [w450 w451] -> w419
          frame "s" {
            w450 = u16 0 items=["Single", "Double"] ("sweep mode")
          }
          frame "d", Default {
            w451 = u16 1 items=["Single", "Double"] ("sweep mode")
          }
        }
        n117 = Fract/Exp String To Number(string=w420) -> (number=w402:dbl[])  [unwired: 3 in, 1 out]
        n118 = String To Path(string=w434) -> (path=w430:path)
        n119 = Index Array(array=w402, index #1=0 ("Index")) -> (element #1=w418:dbl, element #2=w417:dbl, element #3=w416:dbl)  [unwired: 2 in]
        n120 = Delete From Array(array=w402, length=3 ("Length"), index=0 ("Index")) -> (array with subset deleted=w401:dbl[])  [unwired: 1 out]
        n121 = Bundle By Name(cluster=w410, "Gate Start"=w418, "Gate Stop"=w417, "Gate Step (linear only)"=w416, "Gate Compliance"=w428, "Range mode"=w394, "Range"=w393) -> (w448:T3)
        n122 = Index Array(array=w401, index #1=0 ("Index")) -> (element #1=w413:dbl, element #2=w412:dbl, element #3=w411:dbl)  [unwired: 2 in]
        n123 = call <vilib>:"compatOverwrite.vi"("overwrite (F)"=TRUE) -> ("overwrite?"=w385:T7)
        n124 = Bundle By Name(cluster=w409, "Drain Start"=w413, "Drain Stop"=w412, "Drain Step"=w411, "Drain Compliance"=w429, "Range mode"=w392, "Range"=w395) -> (w447:T4)
        n125 = call "4155C Output.vi"("VISA resource name in"=w398, "Gate"=w448, "Drain"=w447, "Timings"=w427, "error in (no error)"=w397, "SMU4"=w387, "sweep mode"=w419, "Panel controls"=w449) -> ("VD"=w435:dbl[], "Outparams"=w390:T8, "VISA Resource Name out"=w425:refnum<visa-resource-name>, "IS"=w438:dbl[], "ID"=w437:dbl[], "IG"=w436:dbl[], "error out"=w426:errorcluster, "SMU4"=w386:dbl[])  [unwired: 12 in]
        n126 = Unbundle By Name(w390) -> ("V2 Step"=w391:dbl, "V2 Start"=w389:dbl, "Number of points"=w388:i32)
        n127 = Open/Create/Replace File(file path (use dialog)=w430, error in=w426, operation (0:open)=w385) -> (refnum out=w444:refnum<file>, error out=w445:errorcluster)  [unwired: 3 in, 1 out]
        n128 = call "4155C Make Big 2d array.vi"("1D Var1"=w435, "1d IS"=w438, "1d ID"=w437, "1d IG"=w436, "1d SMU4"=w386, "SMU4"=w387, "VAR2 START"=w389, "Number of VAR2 steps"=w388, "VAR2 STEP"=w391, "VAR1 Name"="Vd", "Decimal places in header"=i8 1, "VAR2 Name"="Vg") -> ("Header array"=w440:string[], "Data array"=w441:dbl[][])  [unwired: 14 in]
        n129 = call "4155C Write array to file.vi"("Byte Stream File Refnum"=w444, "Header"=w440, "Data Array"=w441, "error in (no error)"=w445) -> ("dup refnum"=w442:refnum<file>, "error out"=w443:errorcluster)  [unwired: 1 in]
        n130 = Close File(refnum=w442, error in=w443) -> (error out=w424:errorcluster)  [unwired: 1 out]
      }
      frame "output-fpp" {
        n131 = Number To Decimal String(number=w453) -> (decimal integer string=w507:string)  [unwired: 1 in]
        n132 = Bundle By Name(cluster=w483, "Emergency Stop"=w510) -> (w520:T6)
        n133 = Delete From Array(array=w498, index=0 ("Index")) -> (deleted portion=w496:string, array with subset deleted=w495:string[])  [unwired: 1 in]
        n134 = VISA Write(VISA resource name=w474, write buffer=":PAGE:CHAN:MODE SWE;" ("write buffer (\"\")"), error in (no error)=w471) -> (VISA resource name out=w473:refnum<visa-resource-name>, error out=w472:errorcluster)  [unwired: 1 out]
        n135 = Concatenate Strings(w506, "-outputfpp-" ("Substring"), w507, w452, ".txt" ("Substring")) -> (w509:string)
        n136 = case shown="\"d\", Default" w496 {
          tunnel: [w521 w522] -> w494
          frame "s" {
            w521 = u16 0 items=["Single", "Double"] ("sweep mode")
          }
          frame "d", Default {
            w522 = u16 1 items=["Single", "Double"] ("sweep mode")
          }
        }
        n137 = Fract/Exp String To Number(string=w495) -> (number=w477:dbl[])  [unwired: 3 in, 1 out]
        n138 = String To Path(string=w509) -> (path=w505:path)
        n139 = Index Array(array=w477, index #1=0 ("Index")) -> (element #1=w493:dbl, element #2=w492:dbl, element #3=w491:dbl)  [unwired: 2 in]
        n140 = Delete From Array(array=w477, length=3 ("Length"), index=0 ("Index")) -> (array with subset deleted=w476:dbl[])  [unwired: 1 out]
        n141 = Bundle By Name(cluster=w485, "Gate Start"=w493, "Gate Stop"=w492, "Gate Step (linear only)"=w491, "Gate Compliance"=w503, "Range mode"=w469, "Range"=w468) -> (w519:T3)
        n142 = Index Array(array=w476, index #1=0 ("Index")) -> (element #1=w488:dbl, element #2=w487:dbl, element #3=w486:dbl)  [unwired: 2 in]
        n143 = call <vilib>:"compatOverwrite.vi"("overwrite (F)"=TRUE) -> ("overwrite?"=w457:T7)
        n144 = Bundle By Name(cluster=w484, "Drain Start"=w488, "Drain Stop"=w487, "Drain Step"=w486, "Drain Compliance"=w504, "Range mode"=w467, "Range"=w470) -> (w518:T4)
        n145 = call "4155C Output-FPP.vi"("VISA resource name in"=w473, "Gate"=w519, "Drain"=w518, "Timings"=w502, "error in (no error)"=w472, "sweep mode"=w494, "Panel controls"=w520) -> ("VD"=w462:dbl[], "Outparams"=w465:T8, "VISA Resource Name out"=w500:refnum<visa-resource-name>, "Vprobe2"=w461:dbl[], "ID"=w460:dbl[], "IG"=w459:dbl[], "Vprobe1"=w458:dbl[], "error out"=w501:errorcluster)  [unwired: 13 in]
        n146 = Unbundle By Name(w465) -> ("V2 Step"=w466:dbl, "V2 Start"=w464:dbl, "Number of points"=w463:i32)
        n147 = Open/Create/Replace File(file path (use dialog)=w505, error in=w501, operation (0:open)=w457) -> (refnum out=w515:refnum<file>, error out=w516:errorcluster)  [unwired: 3 in, 1 out]
        n148 = call "4155C Make Big 2d array FPP.vi"("1D Var1"=w462, "1d ID"=w460, "1d Vp2"=w461, "1d IG"=w459, "1d Vp1"=w458, "VAR2 START"=w464, "Number of VAR2 steps"=w463, "VAR2 STEP"=w466, "VAR1 Name"="Vd", "Decimal places in header"=i8 1, "VAR2 Name"="Vg") -> ("Header array"=w511:string[], "Data array"=w512:dbl[][])  [unwired: 15 in]
        n149 = call "4155C Write array to file.vi"("Byte Stream File Refnum"=w515, "Header"=w511, "Data Array"=w512, "error in (no error)"=w516) -> ("dup refnum"=w513:refnum<file>, "error out"=w514:errorcluster)  [unwired: 1 in]
        n150 = Close File(refnum=w513, error in=w514) -> (error out=w499:errorcluster)  [unwired: 1 out]
      }
      frame "itime" {
        n151 = Delete From Array(array=w536, index=0 ("Index")) -> (deleted portion=w537:string)  [unwired: 1 in, 1 out]
        n152 = case shown="\"l\"" w537 {
          tunnel: w535 -> [w541 w543 w546]
          tunnel: [w540 w542 w545] -> w528
          frame "s" {
            w539 = u32 0 items=["short  ", "medium  ", "long  "] ("integration time 2")
            n153 = Bundle By Name(cluster=w541, "integration time"=w539) -> (w540:T5)
          }
          frame "m", Default {
            w544 = u32 1 items=["short  ", "medium  ", "long  "] ("integration time 2")
            n154 = Bundle By Name(cluster=w543, "integration time"=w544) -> (w542:T5)
          }
          frame "l" {
            w547 = u32 2 items=["short  ", "medium  ", "long  "] ("integration time 2")
            n155 = Bundle By Name(cluster=w546, "integration time"=w547) -> (w545:T5)
          }
        }
      }
      frame "pulsed" {
        n156 = Delete From Array(array=w562, index=0 ("Index")) -> (deleted portion=w563:string, array with subset deleted=w550:string[])  [unwired: 1 in]
        n157 = case shown="\"on\", Default" w563 {
          tunnel: w561 -> [w573 w576]
          tunnel: [w572 w575] -> w554
          tunnel: w550 -> [w570 _]
          frame "on", Default {
            w571 = u16 1 items=["Continuous", "Pulsed"] ("sweep method")
            n158 = Fract/Exp String To Number(string=w570) -> (number=w568:dbl[])  [unwired: 3 in, 1 out]
            n159 = Index Array(array=w568, index #1=0 ("Index")) -> (element #1=w567:dbl, element #2=w566:dbl, element #3=w565:dbl)  [unwired: 2 in]
            n160 = Bundle By Name(cluster=w573, "sweep method"=w571, "Pulse period"=w567, "Base voltage"=w566, "Pulse width"=w565) -> (w572:T5)
          }
          frame "off" {
            w574 = u16 0 items=["Continuous", "Pulsed"] ("sweep method")
            n161 = Bundle By Name(cluster=w576, "sweep method"=w574) -> (w575:T5)
          }
        }
      }
      frame "gaterangemode" {
        n162 = Delete From Array(array=w589, index=0 ("Index")) -> (deleted portion=w590:string)  [unwired: 1 in, 1 out]
        n163 = case shown="\"f\"" w590 {
          tunnel: [w592 w593 w594] -> w579
          frame "a", Default {
            w592 = u16 0 items=["Auto", "Limited", "Fixed"] ("Gate Range\nmode 2")
          }
          frame "f" {
            w593 = u16 2 items=["Auto", "Limited", "Fixed"] ("Gate Range\nmode 2")
          }
          frame "l" {
            w594 = u16 1 items=["Auto", "Limited", "Fixed"] ("Gate Range\nmode 2")
          }
        }
      }
      frame "gaterange" {
        (unwired) u8 11 items=["10fA  ", "100fA  ", "1nA  ", "10nA", "100nA", "1uA", "10uA", "100uA", "1mA", "10mA", "100mA", "1A"] ("Gate Range 2")
        n164 = Delete From Array(array=w614, index=0 ("Index")) -> (deleted portion=w604:string)  [unwired: 1 in, 1 out]
        n165 = Scan Value(string=w604, format string="") -> (value=w602:dbl)  [unwired: 1 in, 1 out]
        n166 = Logarithm Base 10(1:w602) -> (0:w601:dbl)
        n167 = Round To Nearest(number=w601) -> (nearest integer value=w600:dbl)
        n168 = Add(x=w600, y=11.0) -> (x+y=w598:dbl)
        n169 = To Unsigned Byte Integer(number=w598) -> (unsigned 8bit integer=w597:u8)
      }
      frame "drainrange" {
        (unwired) u8 11 items=["10fA  ", "100fA  ", "1nA  ", "10nA", "100nA", "1uA", "10uA", "100uA", "1mA", "10mA", "100mA", "1A"] ("Gate Range 2")
        n170 = Delete From Array(array=w635, index=0 ("Index")) -> (deleted portion=w626:string)  [unwired: 1 in, 1 out]
        n171 = Scan Value(string=w626, format string="") -> (value=w624:dbl)  [unwired: 1 in, 1 out]
        n172 = Logarithm Base 10(1:w624) -> (0:w623:dbl)
        n173 = Round To Nearest(number=w623) -> (nearest integer value=w622:dbl)
        n174 = Add(x=w622, y=11.0) -> (x+y=w620:dbl)
        n175 = To Unsigned Byte Integer(number=w620) -> (unsigned 8bit integer=w619:u8)
      }
      frame "drainrangemode" {
        n176 = Delete From Array(array=w649, index=0 ("Index")) -> (deleted portion=w650:string)  [unwired: 1 in, 1 out]
        n177 = case shown="\"f\"" w650 {
          tunnel: [w652 w653 w654] -> w639
          frame "a", Default {
            w652 = u16 0 items=["Auto", "Limited", "Fixed"] ("Gate Range\nmode 2")
          }
          frame "f" {
            w653 = u16 2 items=["Auto", "Limited", "Fixed"] ("Gate Range\nmode 2")
          }
          frame "l" {
            w654 = u16 1 items=["Auto", "Limited", "Fixed"] ("Gate Range\nmode 2")
          }
        }
      }
      frame "Error", Default {
      }
      frame "logfile" {
        n178 = Number To Decimal String(number=w669) -> (decimal integer string=w704:string)  [unwired: 1 in]
        n179 = Concatenate Strings(w703, "logfile" ("Substring"), w704, w667, ".txt" ("Substring")) -> (w701:string)
        n180 = String To Path(string=w701) -> (path=w674:path)
        n181 = Unbundle(w700) -> ("integration time"=w699:u32, "Short/Long integration time"=w698:dbl, "hold time (sec)"=w697:dbl, "delay time (sec)"=w696:dbl, "Step Time (0 disables)"=w695:dbl, "sweep method"=w694:u16, "Pulse period"=w693:dbl, "Base voltage"=w692:dbl, "Pulse width"=w691:dbl)
        n182 = Build Array(w699, w698, w697, w696, w695, w694, w693, w692, w691, w685, w686, w687, w688, w689, w690) -> (w678:dbl[])
        n183 = Insert Into Array(array=dbl[][] [] ("Input Array"), new element=w678) -> (w677:dbl[][])  [unwired: 2 in]
        n184 = call <vilib>:"compatOverwrite.vi"("overwrite (F)"=TRUE) -> ("overwrite?"=w672:T7)
        n185 = Open/Create/Replace File(file path (use dialog)=w674, error in=w676, operation (0:open)=w672) -> (refnum out=w682:refnum<file>, error out=w681:errorcluster)  [unwired: 3 in, 1 out]
        n186 = call "4155C Write array to file.vi"("Byte Stream File Refnum"=w682, "Header"=string[] ["Int Time", "Short/Long Itime", "Hold time", "Delay time", "Step time", "Sweep method", "Pulse period", "Base Voltage", "Pulse width", "Drain compliance", "Gate compliance", "Gate range mode", "Gate range", "S/D range mode", "S/D range"], "Data Array"=w677, "error in (no error)"=w681) -> ("dup refnum"=w684:refnum<file>, "error out"=w683:errorcluster)  [unwired: 1 in]
        n187 = Close File(refnum=w684, error in=w683) -> (error out=w675:errorcluster)  [unwired: 1 out]
      }
      frame "sample" {
        n188 = Number To Decimal String(number=w708) -> (decimal integer string=w756:string)  [unwired: 1 in]
        n189 = Fract/Exp String To Number(string=w753) -> (number=w714:dbl[])  [unwired: 3 in, 1 out]
        n190 = Concatenate Strings(w731, "-sample-" ("Substring"), w756, w706, ".txt" ("Substring")) -> (w754:string)
        n191 = String To Path(string=w754) -> (path=w735:path)
        n192 = Index Array(array=w714, index=0 ("Index")) -> (element=w751:dbl)
        n193 = Index Array(array=w714, index=2 ("Index")) -> (element=w747:dbl)
        n194 = Index Array(array=w714, index=3 ("Index")) -> (element=w716:dbl)
        n195 = Index Array(array=w714, index=4 ("Index")) -> (element=w713:dbl)
        n196 = call "4155C Config Sampling Measurements.vi"("Sampling interval"=w713, "Sample time"=w716, "Display on/off"=TRUE, "Timings"=w722, "Num Points"=w747, "error in (no error)"=w758, "Drain Compliance"=w757, "Gate Compliance"=w732, "VISA session"=w759) -> ("error out"=w760:errorcluster, "dup VISA resource name"=w761:refnum<visa-resource-name>)  [unwired: 1 in]
        n197 = Index Array(array=w714, index=1 ("Index")) -> (element=w748:dbl)
        n198 = call "4155C Take Sample.vi"("Emergency Stop"=w728, "error in (no error)"=w760, "Vd"=w748, "Vg"=w751, "VISA resource name in"=w761) -> ("error out"=w726:errorcluster, "Id"=w763:dbl[], "Ig"=w737:dbl[], "VISA Resource Name out"=w724:refnum<visa-resource-name>, "Is"=w762:dbl[], "Time"=w741:dbl[])  [unwired: 1 in]
        n199 = Insert Into Array(array=dbl[][] [] ("Input Array"), new element=w741) -> (w740:dbl[][])  [unwired: 2 in]
        n200 = Insert Into Array(array=w740, new element=w737) -> (w739:dbl[][])  [unwired: 2 in]
        n201 = Insert Into Array(array=w739, new element=w763) -> (w738:dbl[][])  [unwired: 2 in]
        n202 = VISA Write(VISA resource name=w724, write buffer=":DISP ON" ("write buffer (\"\")"), error in (no error)=w726) -> (VISA resource name out=w723:refnum<visa-resource-name>, error out=w725:errorcluster)  [unwired: 1 out]
        n203 = Insert Into Array(array=w738, new element=w762) -> (w730:dbl[][])  [unwired: 2 in]
        n204 = Transpose 2D Array(2D array=w730) -> (transposed array=w729:dbl[][])
        n205 = call <vilib>:"compatOverwrite.vi"("overwrite (F)"=TRUE) -> ("overwrite?"=w711:T7)
        n206 = Open/Create/Replace File(file path (use dialog)=w735, error in=w725, operation (0:open)=w711) -> (refnum out=w744:refnum<file>, error out=w743:errorcluster)  [unwired: 3 in, 1 out]
        n207 = call "4155C Write array to file.vi"("Byte Stream File Refnum"=w744, "Header"=string[] ["Time /s", "Ig /A", "Id /A", "Is /A"], "Data Array"=w729, "error in (no error)"=w743) -> ("dup refnum"=w746:refnum<file>, "error out"=w745:errorcluster)  [unwired: 1 in]
        n208 = Close File(refnum=w746, error in=w745) -> (error out=w733:errorcluster)  [unwired: 1 out]
      }
      frame "samplei" {
        n209 = Number To Decimal String(number=w765) -> (decimal integer string=w817:string)  [unwired: 1 in]
        n210 = Fract/Exp String To Number(string=w814) -> (number=w781:dbl[])  [unwired: 3 in, 1 out]
        n211 = Concatenate Strings(w796, "-samplei-" ("Substring"), w817, w764, ".txt" ("Substring")) -> (w815:string)
        n212 = String To Path(string=w815) -> (path=w799:path)
        n213 = Index Array(array=w781, index=4 ("Index")) -> (element=w775:dbl)
        n214 = Index Array(array=w781, index=3 ("Index")) -> (element=w776:dbl)
        n215 = Index Array(array=w781, index=1 ("Index")) -> (element=w778:dbl)
        n216 = Index Array(array=w781, index=0 ("Index")) -> (element=w779:dbl)
        n217 = Index Array(array=w781, index=2 ("Index")) -> (element=w777:dbl)
        n218 = call "4155C Config SamplingI Measurements.vi"("Sample time"=w777, "Display on/off"=TRUE, "Timings"=w788, "Num Points"=w778, "error in (no error)"=w819, "Sampling interval"=w776, "VISA session"=w820) -> ("error out"=w821:errorcluster, "dup VISA resource name"=w822:refnum<visa-resource-name>)  [unwired: 3 in]
        n219 = call "4155C Take SampleI.vi"("Emergency Stop"=w793, "error in (no error)"=w821, "Idg 2"=w779, "Vdg compliance 2"=w775, "VISA resource name in"=w822) -> ("error out"=w791:errorcluster, "Idg"=w824:dbl[], "Vdg"=w801:dbl[], "VISA Resource Name out"=w789:refnum<visa-resource-name>, "Is"=w823:dbl[], "Time"=w805:dbl[])  [unwired: 1 in]
        n220 = Insert Into Array(array=dbl[][] [] ("Input Array"), new element=w805) -> (w804:dbl[][])  [unwired: 2 in]
        n221 = Insert Into Array(array=w804, new element=w801) -> (w803:dbl[][])  [unwired: 2 in]
        n222 = Insert Into Array(array=w803, new element=w824) -> (w802:dbl[][])  [unwired: 2 in]
        n223 = VISA Write(VISA resource name=w789, write buffer=":DISP ON" ("write buffer (\"\")"), error in (no error)=w791) -> (VISA resource name out=w774:refnum<visa-resource-name>, error out=w790:errorcluster)  [unwired: 1 out]
        n224 = Insert Into Array(array=w802, new element=w823) -> (w795:dbl[][])  [unwired: 2 in]
        n225 = Transpose 2D Array(2D array=w795) -> (transposed array=w794:dbl[][])
        n226 = call <vilib>:"compatOverwrite.vi"("overwrite (F)"=TRUE) -> ("overwrite?"=w769:T7)
        n227 = Open/Create/Replace File(file path (use dialog)=w799, error in=w790, operation (0:open)=w769) -> (refnum out=w808:refnum<file>, error out=w807:errorcluster)  [unwired: 3 in, 1 out]
        n228 = call "4155C Write array to file.vi"("Byte Stream File Refnum"=w808, "Header"=string[] ["Time /s", "Vdg /V", "Idg /A", "Is /A"], "Data Array"=w794, "error in (no error)"=w807) -> ("dup refnum"=w810:refnum<file>, "error out"=w809:errorcluster)  [unwired: 1 in]
        n229 = Close File(refnum=w810, error in=w809) -> (error out=w772:errorcluster)  [unwired: 1 out]
        n230 = VISA Write(VISA resource name=w774, write buffer=";:PAGE:SCON:STAN OFF;:PAGE:CHAN:VSU2:DIS;" ("write buffer (\"\")"), error in (no error)=w772) -> (VISA resource name out=w770:refnum<visa-resource-name>, error out=w771:errorcluster)  [unwired: 1 out]
      }
      frame "#" {
        n231 = VISA Write(VISA resource name=w831, write buffer=":DISP ON" ("write buffer (\"\")"), error in (no error)=w830) -> (VISA resource name out=w829:refnum<visa-resource-name>, error out=w828:errorcluster)  [unwired: 1 out]
      }
      frame "stressV" {
        n232 = Number To Decimal String(number=w841) -> (decimal integer string=w882:string)  [unwired: 1 in]
        n233 = Fract/Exp String To Number(string=w879) -> (number=w852:dbl[])  [unwired: 3 in, 1 out]
        n234 = Concatenate Strings(w866, "-stressV-" ("Substring"), w882, w840, ".txt" ("Substring")) -> (w880:string)
        n235 = String To Path(string=w880) -> (path=w870:path)
        n236 = Index Array(array=w852, index=3 ("Index")) -> (element=w849:dbl)
        n237 = Index Array(array=w852, index=1 ("Index")) -> (element=w847:dbl)
        n238 = Index Array(array=w852, index=0 ("Index")) -> (element=w846:dbl)
        n239 = Index Array(array=w852, index=4 ("Index")) -> (element=w851:dbl)
        n240 = Index Array(array=w852, index=2 ("Index")) -> (element=w848:dbl)
        n241 = call "4155C Config V Stress.vi"("VISA session"=w885, "ID compliance"=w849, "VD"=w847, "VG"=w846, "IG compliance"=w848, "error in (no error)"=w884, "Display on/off"=TRUE) -> ("dup VISA resource name"=w887:refnum<visa-resource-name>, "error out"=w886:errorcluster)
        n242 = call "4155C Apply Stress.vi"("error in (no error)"=w886, "Duration"=w851, "Emergency Stop"=w865, "VISA resource name in"=w887) -> ("error out"=w863:errorcluster, "VISA Resource Name out"=w861:refnum<visa-resource-name>)
        n243 = VISA Write(VISA resource name=w861, write buffer=":DISP ON" ("write buffer (\"\")"), error in (no error)=w863) -> (VISA resource name out=w860:refnum<visa-resource-name>, error out=w862:errorcluster)  [unwired: 1 out]
        n244 = call <vilib>:"compatOverwrite.vi"("overwrite (F)"=TRUE) -> ("overwrite?"=w845:T7)
        n245 = Open/Create/Replace File(file path (use dialog)=w870, error in=w862, operation (0:open)=w845) -> (refnum out=w873:refnum<file>, error out=w872:errorcluster)  [unwired: 3 in, 1 out]
        n246 = call "4155C Write array to file.vi"("Byte Stream File Refnum"=w873, "Header"=string[] ["V stress completed successfully", ""], "error in (no error)"=w872) -> ("dup refnum"=w875:refnum<file>, "error out"=w874:errorcluster)  [unwired: 2 in]
        n247 = Close File(refnum=w875, error in=w874) -> (error out=w868:errorcluster)  [unwired: 1 out]
      }
      frame "stressI" {
        n248 = Number To Decimal String(number=w889) -> (decimal integer string=w926:string)  [unwired: 1 in]
        n249 = Fract/Exp String To Number(string=w923) -> (number=w898:dbl[])  [unwired: 3 in, 1 out]
        n250 = Concatenate Strings(w910, "-stressI-" ("Substring"), w926, w888, ".txt" ("Substring")) -> (w924:string)
        n251 = String To Path(string=w924) -> (path=w914:path)
        n252 = Index Array(array=w898, index=1 ("Index")) -> (element=w894:dbl)
        n253 = Index Array(array=w898, index=0 ("Index")) -> (element=w895:dbl)
        n254 = call "4155C Config I Stress.vi"("VISA session"=w929, "IDG"=w895, "VDG compliance"=w894, "error in (no error)"=w928, "Display on/off"=TRUE) -> ("dup VISA resource name"=w931:refnum<visa-resource-name>, "error out"=w930:errorcluster)
        n255 = Index Array(array=w898, index=2 ("Index")) -> (element=w896:dbl)
        n256 = call "4155C Apply Stress.vi"("error in (no error)"=w930, "Duration"=w896, "Emergency Stop"=w909, "VISA resource name in"=w931) -> ("error out"=w907:errorcluster, "VISA Resource Name out"=w905:refnum<visa-resource-name>)
        n257 = VISA Write(VISA resource name=w905, write buffer=":DISP ON" ("write buffer (\"\")"), error in (no error)=w907) -> (VISA resource name out=w904:refnum<visa-resource-name>, error out=w906:errorcluster)  [unwired: 1 out]
        n258 = call <vilib>:"compatOverwrite.vi"("overwrite (F)"=TRUE) -> ("overwrite?"=w893:T7)
        n259 = Open/Create/Replace File(file path (use dialog)=w914, error in=w906, operation (0:open)=w893) -> (refnum out=w917:refnum<file>, error out=w916:errorcluster)  [unwired: 3 in, 1 out]
        n260 = call "4155C Write array to file.vi"("Byte Stream File Refnum"=w917, "Header"=string[] ["I stress completed successfully", ""], "error in (no error)"=w916) -> ("dup refnum"=w919:refnum<file>, "error out"=w918:errorcluster)  [unwired: 2 in]
        n261 = Close File(refnum=w919, error in=w918) -> (error out=w912:errorcluster)  [unwired: 1 out]
      }
      frame "vsu2pulse" {
        n262 = Number To Decimal String(number=w933) -> (decimal integer string=w968:string)  [unwired: 1 in]
        n263 = Fract/Exp String To Number(string=w965) -> (number=w941:dbl[])  [unwired: 3 in, 1 out]
        n264 = Concatenate Strings(w953, "-vsu2-" ("Substring"), w968, w932, ".txt" ("Substring")) -> (w966:string)
        n265 = String To Path(string=w966) -> (path=w957:path)
        n266 = Index Array(array=w941, index=1 ("Index")) -> (element=w940:dbl)
        n267 = Index Array(array=w941, index=0 ("Index")) -> (element=w938:dbl)
        n268 = call "4155C Config VSU2 Stress.vi"("error in (no error)"=w970, "VSU2"=w938, "Display on/off"=TRUE, "VISA session"=w971) -> ("error out"=w972:errorcluster, "dup VISA resource name"=w973:refnum<visa-resource-name>)
        n269 = call "4155C Apply Stress.vi"("error in (no error)"=w972, "Duration"=w940, "Emergency Stop"=w952, "VISA resource name in"=w973) -> ("error out"=w950:errorcluster, "VISA Resource Name out"=w948:refnum<visa-resource-name>)
        n270 = VISA Write(VISA resource name=w948, write buffer=":DISP ON" ("write buffer (\"\")"), error in (no error)=w950) -> (VISA resource name out=w947:refnum<visa-resource-name>, error out=w949:errorcluster)  [unwired: 1 out]
        n271 = call <vilib>:"compatOverwrite.vi"("overwrite (F)"=TRUE) -> ("overwrite?"=w937:T7)
        n272 = Open/Create/Replace File(file path (use dialog)=w957, error in=w949, operation (0:open)=w937) -> (refnum out=w960:refnum<file>, error out=w959:errorcluster)  [unwired: 3 in, 1 out]
        n273 = call "4155C Write array to file.vi"("Byte Stream File Refnum"=w960, "Header"=string[] ["VSU2 pulse completed successfully", ""], "error in (no error)"=w959) -> ("dup refnum"=w962:refnum<file>, "error out"=w961:errorcluster)  [unwired: 2 in]
        n274 = Close File(refnum=w962, error in=w961) -> (error out=w955:errorcluster)  [unwired: 1 out]
      }
      frame "sample-fpp" {
        w986 = string[] ["Time /s", "Id VgVd /A", "Ig VgVd /A", "Vp1 VgVd /V", "Vp2 VgVd /V"] ("Header")
        w990 = "%d" ("format string")
        n275 = Number To Decimal String(number=w975) -> (decimal integer string=w1038:string)  [unwired: 1 in]
        n276 = Fract/Exp String To Number(string=w1035) -> (number=w1023:dbl[])  [unwired: 3 in, 1 out]
        n277 = Concatenate Strings(w1029, "-samplefpp-" ("Substring"), w1038, w974, ".txt" ("Substring")) -> (w1036:string)
        n278 = String To Path(string=w1036) -> (path=w998:path)
        n279 = Index Array(array=w1023, index=0 ("Index")) -> (element=w984:dbl)
        n280 = Index Array(array=w1023, index=1 ("Index")) -> (element=w983:dbl)
        n281 = Index Array(array=w1023, index=2 ("Index")) -> (element=w1031:dbl)
        n282 = Index Array(array=w1023, index=3 ("Index")) -> (element=w1021:dbl)
        n283 = call "4155C Config Sampling Measurements FPP.vi"("VISA session"=w1041, "Num Points"=w1031, "Vg"=w984, "Display on/off"=TRUE, "Gate Compliance"=w1030, "Drain Compliance"=w1039, "Standby"="Standby", "error in (no error)"=w1040, "Timings"=w1028, "Vd"=w983, "Sample time"=w1021) -> ("dup VISA resource name"=w1000:refnum<visa-resource-name>, "error out"=w999:errorcluster)  [unwired: 3 in]
        n284 = Number To Decimal String(number=w984) -> (decimal integer string=w1010:string)  [unwired: 1 in]
        n285 = call "4155C Take Sample FPP.vi"("VISA resource name in"=w1000, "error in (no error)"=w999, "Emergency Stop"=w1001) -> ("Time"=w1005:dbl[], "Vp1"=w1015:dbl[], "VISA Resource Name out"=w981:refnum<visa-resource-name>, "Ig"=w1003:dbl[], "Id"=w1004:dbl[], "Vp2"=w1013:dbl[], "error out"=w1002:errorcluster)  [unwired: 10 in]
        n286 = Insert Into Array(array=dbl[][] [] ("Input Array"), new element=w1005) -> (w1019:dbl[][])  [unwired: 2 in]
        n287 = Number To Decimal String(number=w983) -> (decimal integer string=w1008:string)  [unwired: 1 in]
        n288 = Insert Into Array(array=w1019, new element=w1004) -> (w1018:dbl[][])  [unwired: 2 in]
        n289 = Concatenate Strings("(Vg = " ("Substring"), w1010, "V, Vd = " ("Substring"), w1008, "V)" ("Substring")) -> (w1006:string)
        n290 = Insert Into Array(array=w1018, new element=w1003) -> (w1017:dbl[][])  [unwired: 2 in]
        n291 = Insert Into Array(array=w1017, new element=w1015) -> (w1014:dbl[][])  [unwired: 2 in]
        n292 = Insert Into Array(array=w1014, new element=w1013) -> (w982:dbl[][])  [unwired: 2 in]
        n293 = call <vilib>:"compatOverwrite.vi"("overwrite (F)"=TRUE) -> ("overwrite?"=w979:T7)
        n294 = Open/Create/Replace File(file path (use dialog)=w998, error in=w1002, operation (0:open)=w979) -> (refnum out=w995:refnum<file>, error out=w996:errorcluster)  [unwired: 3 in, 1 out]
        n295 = Array To Spreadsheet String(array=w986, 3:w990) -> (spreadsheet string=w992:string)  [unwired: 1 in]
        n296 = Transpose 2D Array(2D array=w982) -> (transposed array=w1012:dbl[][])
        n297 = Search and Replace String(replace all?=TRUE ("replace all? (F)"), input string=w992, search string="VgVd", replace string=w1006) -> (result string=w988:string)  [unwired: 4 in, 3 out]
        n298 = Spreadsheet String To Array(format string=w990, spreadsheet string=w988, array type (2D Dbl)=w986) -> (array=w987:string[])  [unwired: 1 in]
        n299 = call "4155C Write array to file.vi"("Byte Stream File Refnum"=w995, "Header"=w987, "Data Array"=w1012, "error in (no error)"=w996) -> ("dup refnum"=w993:refnum<file>, "error out"=w994:errorcluster)  [unwired: 1 in]
        n300 = Close File(refnum=w993, error in=w994) -> (error out=w980:errorcluster)  [unwired: 1 out]
      }
      frame "resample-fpp" {
        w1056 = string[] ["Time /s", "Id VgVd /A", "Ig VgVd /A", "Vp1 VgVd /V", "Vp2 VgVd /V"] ("Header")
        w1060 = "%d" ("format string")
        n301 = Number To Decimal String(number=w1042) -> (decimal integer string=w1100:string)  [unwired: 1 in]
        n302 = Fract/Exp String To Number(string=w1097) -> (number=w1049:dbl[])  [unwired: 3 in, 1 out]
        n303 = Concatenate Strings(w1093, "-resamplefpp-" ("Substring"), w1100, w1043, ".txt" ("Substring")) -> (w1098:string)
        n304 = String To Path(string=w1098) -> (path=w1068:path)
        n305 = Index Array(array=w1049, index=0 ("Index")) -> (element=w1055:dbl)
        n306 = Index Array(array=w1049, index=1 ("Index")) -> (element=w1054:dbl)
        n307 = Number To Decimal String(number=w1055) -> (decimal integer string=w1078:string)  [unwired: 1 in]
        n308 = call "4155C Take Sample FPP.vi"("VISA resource name in"=w1051, "error in (no error)"=w1050, "Emergency Stop"=w1069) -> ("Time"=w1073:dbl[], "Vp1"=w1083:dbl[], "VISA Resource Name out"=w1053:refnum<visa-resource-name>, "Ig"=w1071:dbl[], "Id"=w1072:dbl[], "Vp2"=w1081:dbl[], "error out"=w1070:errorcluster)  [unwired: 10 in]
        n309 = Insert Into Array(array=dbl[][] [] ("Input Array"), new element=w1073) -> (w1087:dbl[][])  [unwired: 2 in]
        n310 = Number To Decimal String(number=w1054) -> (decimal integer string=w1076:string)  [unwired: 1 in]
        n311 = Insert Into Array(array=w1087, new element=w1072) -> (w1086:dbl[][])  [unwired: 2 in]
        n312 = Concatenate Strings("(Vg = " ("Substring"), w1078, "V, Vd = " ("Substring"), w1076, "V)" ("Substring")) -> (w1074:string)
        n313 = Insert Into Array(array=w1086, new element=w1071) -> (w1085:dbl[][])  [unwired: 2 in]
        n314 = Insert Into Array(array=w1085, new element=w1083) -> (w1082:dbl[][])  [unwired: 2 in]
        n315 = Insert Into Array(array=w1082, new element=w1081) -> (w1048:dbl[][])  [unwired: 2 in]
        n316 = call <vilib>:"compatOverwrite.vi"("overwrite (F)"=TRUE) -> ("overwrite?"=w1047:T7)
        n317 = Open/Create/Replace File(file path (use dialog)=w1068, error in=w1070, operation (0:open)=w1047) -> (refnum out=w1065:refnum<file>, error out=w1066:errorcluster)  [unwired: 3 in, 1 out]
        n318 = Array To Spreadsheet String(array=w1056, 3:w1060) -> (spreadsheet string=w1062:string)  [unwired: 1 in]
        n319 = Transpose 2D Array(2D array=w1048) -> (transposed array=w1080:dbl[][])
        n320 = Search and Replace String(replace all?=TRUE ("replace all? (F)"), input string=w1062, search string="VgVd", replace string=w1074) -> (result string=w1058:string)  [unwired: 4 in, 3 out]
        n321 = Spreadsheet String To Array(format string=w1060, spreadsheet string=w1058, array type (2D Dbl)=w1056) -> (array=w1057:string[])  [unwired: 1 in]
        n322 = call "4155C Write array to file.vi"("Byte Stream File Refnum"=w1065, "Header"=w1057, "Data Array"=w1080, "error in (no error)"=w1066) -> ("dup refnum"=w1063:refnum<file>, "error out"=w1064:errorcluster)  [unwired: 1 in]
        n323 = Close File(refnum=w1063, error in=w1064) -> (error out=w1052:errorcluster)  [unwired: 1 out]
      }
      frame "serial" {
        n324 = Index Array(array=w1104, index=0 ("Index")) -> (element=w1103:string)
        n325 = call "Serial write and read v0.4.vi"("Termination char\n(0xA = '\\n' = LF)\n(0xD = '\\r' = CR)"="Termination char\n(0xA = '\\n' = LF)\n(0xD = '\\r' = CR)", "Enable Termination\nChar (T)"="Enable Termination\nChar (T)", "parity"="parity", "stop bits"="stop bits", "string to write"=w1103, "flow control"="flow control", "byte count"="byte count", "Serial Settings:Serial End Mode for Reads"="Serial Settings:Serial End Mode for Reads", "Timeout (ms)"="Timeout (ms)", "error in (no error)"=w1109, "VISA resource name"="VISA resource name", "baud rate"="baud rate", "data bits"="data bits") -> ("read string"=→"Serial output":string, "error out"=w1108:errorcluster)  [unwired: 1 in]
      }
    }
    "Line running" <- w54
    "Total lines" <- w53
  }
  "error out" <- w13
